vi "test-rotation3d.vi"(8 "error in (no error)":errorcluster) -> (0 "error out":errorcluster, 3 "ALL TESTS PASSED":bool)   [LabVIEW 2019]
uses:
  <vilib>/Rock Robotics/WPI/ThirdParty/JAS_Junk/TrajLib/TypeDef/ROTATION3D.ctl
  <vilib>/Rock Robotics/WPI/ThirdParty/JAS_Junk/TrajLib/TypeDef/QUATERNION.ctl
  <vilib>/Rock Robotics/WPI/ThirdParty/JAS_Junk/TrajLib/VI/Quaternion_New_Default.vi
  <vilib>/Rock Robotics/WPI/ThirdParty/JAS_Junk/TrajLib/MatBuilder_Create.vi
  <vilib>/Rock Robotics/WPI/ThirdParty/JAS_Junk/TrajLib/VI/Vector_Norm.vi
  <vilib>/Rock Robotics/WPI/ThirdParty/JAS_Junk/TrajLib/VI/Quaternion_New.vi
  <vilib>/Rock Robotics/WPI/ThirdParty/JAS_Junk/TrajLib/VecBuilder_ArrayBy1Fill.vi
  <vilib>/Rock Robotics/WPI/ThirdParty/JAS_Junk/TrajLib/VI/Quaternion_Equals.vi
  <vilib>/Rock Robotics/WPI/ThirdParty/JAS_Junk/TrajLib/VI/Vector_Dot.vi
  <vilib>/Rock Robotics/WPI/ThirdParty/JAS_Junk/TrajLib/VI/Rotation3d_Create_Quaternion.vi
  <vilib>/Analysis/7linalg.llb/QR Decomposition.vi
  <vilib>/Analysis/7linalg.llb/Real QR Decomposition.vi
  <vilib>/Rock Robotics/WPI/ThirdParty/JAS_Junk/TrajLib/Matrix_Transpose.vi
  <vilib>/Analysis/baseanly.llb/A x B.vi
  <vilib>/Analysis/baseanly.llb/Real A x B.vi
  <vilib>/Analysis/baseanly.llb/Determinant.vi
  <vilib>/Analysis/baseanly.llb/Real Determinant.vi
  <vilib>/Rock Robotics/WPI/ThirdParty/JAS_Junk/TrajLib/Matrix_NormF.vi
  <vilib>/Rock Robotics/WPI/ThirdParty/JAS_Junk/TrajLib/MatrixHelper_CoerceSize.vi
  <vilib>/Rock Robotics/WPI/ThirdParty/JAS_Junk/TrajLib/VI/Rotation3d_Times.vi
  <vilib>/Rock Robotics/WPI/ThirdParty/JAS_Junk/TrajLib/MathUtil_Clamp.vi
  <vilib>/Rock Robotics/WPI/ThirdParty/JAS_Junk/TrajLib/Util_CalcDist.vi
  <vilib>/Rock Robotics/WPI/ThirdParty/JAS_Junk/TrajLib/VI/Quaternion_Get_Vect.vi
  <vilib>/Rock Robotics/WPI/ThirdParty/JAS_Junk/TrajLib/VI/Quaternion_Get_W.vi
  <vilib>/Rock Robotics/WPI/ThirdParty/JAS_Junk/TrajLib/VI/Rotation3d_UnaryMinus.vi
  <vilib>/Rock Robotics/WPI/ThirdParty/JAS_Junk/TrajLib/VI/Quaternion_Times.vi
  <vilib>/Rock Robotics/WPI/ThirdParty/JAS_Junk/TrajLib/VI/Quaternion_Normalize.vi
  <vilib>/Analysis/_algsub.llb/Matrix Norm.vi
  <vilib>/Analysis/_algsub.llb/Real Matrix Norm.vi
  <vilib>/Rock Robotics/WPI/ThirdParty/JAS_Junk/TrajLib/VI/Quaternion_Inverse.vi
  <vilib>/Analysis/Matrix/Numeric/Conversions/Array To Matrix - RA.vi
  <vilib>/Analysis/7linalg.llb/Create Special Matrix.vi
  <vilib>/Analysis/7linalg.llb/Create Special Real Matrix.vi
  <vilib>/Analysis/Matrix/Numeric/Subtract/Subtract.vi
  <vilib>/Analysis/Matrix/Numeric/Subtract/Subtract - RM,RM.vi
  <vilib>/Analysis/Matrix/Numeric/Multiply/Multiply - RM,R.vi
  <vilib>/Rock Robotics/WPI/ThirdParty/JAS_Junk/TrajLib/Trajectory_Library.lvlib
  <vilib>/Analysis/Matrix/NI_Matrix.lvlib
panel:
  out "Axis Angle\nTest Passed":bool
  out "Two Vectors\nTest Passed":bool
  out "Rotation3d 2":T1={"Q_quaternion"={"R"=1.0, "V"=[0.0, 0.0, 0.0]}}
  out "Rotation3d":T1={"Q_quaternion"={"R"=1.0, "V"=[0.0, 0.0, 0.0]}}
  out "Rot Mat\nTest Passed":bool
  # "ROTATION3D TEST"
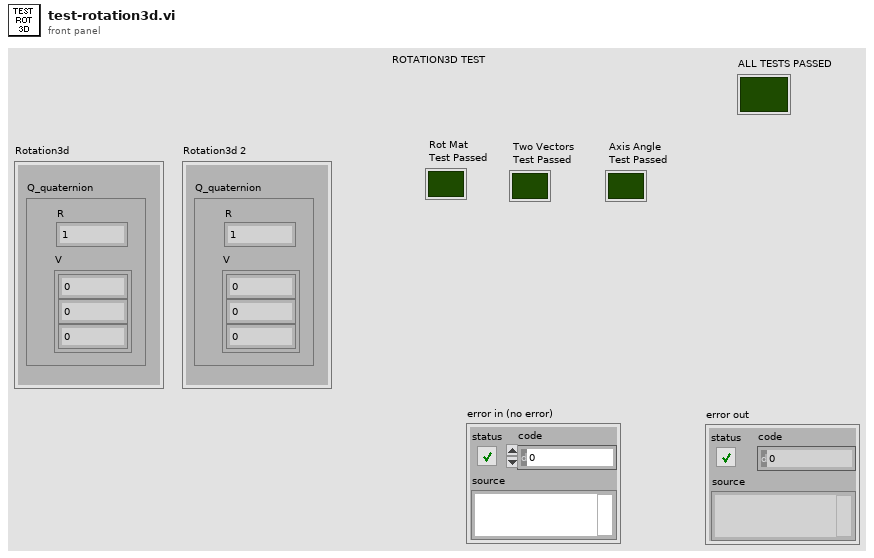
[diagram p1: front panel]
types:
  T1 = typedef "Trajectory_Library.lvlib/ROTATION3D.ctl" = cluster{"Q_quaternion":T2}
  T2 = typedef "Trajectory_Library.lvlib/QUATERNION.ctl" = cluster{"R":dbl, "V":dbl[]}
  T3 = typedef "NI_Matrix.lvlib/RealMatrix.ctl" = dbl[][]
  T4 = typedef "Trajectory_Library.lvlib/ROTATION2D.ctl" = cluster{"VALUE":dbl, "COS":dbl, "SIN":dbl}
diagram:
  w17 = 1.0  # R2
  w16 = 0.0  # R1
  w15 = 0.0  # R0
  w21 = 0.0  # R2
  w20 = 1.0  # R1
  w19 = 0.0  # R0
  w27 = 0.0  # R2
  w26 = 0.0  # R1
  w25 = 1.0  # R0
  w32 = 0.0  # Roll  Degrees
  w33 = 0.0  # Pitch  Degrees
  w34 = 60.0  # Yaw  Degrees
  w43 = 60.0  # Angle Degrees
  w41 = 1.0  # Z
  w39 = 0.0  # X
  w40 = 0.0  # Y
  w45 = 0.0  # Roll  Degrees
  w46 = 60.0  # Pitch  Degrees
  w47 = 0.0  # Yaw  Degrees
  w56 = 60.0  # Angle Degrees
  w54 = 0.0  # Z
  w52 = 0.0  # X
  w53 = 1.0  # Y
  w59 = 60.0  # Roll  Degrees
  w60 = 0.0  # Pitch  Degrees
  w61 = 0.0  # Yaw  Degrees
  w70 = 60.0  # Angle Degrees
  w68 = 0.0  # Z
  w66 = 1.0  # X
  w67 = 0.0  # Y
  w169 = 0.0  # z
  w168 = 1.0  # y
  w167 = 1.0  # x
  w181 = 1.0  # z
  w180 = 0.0  # y
  w179 = 0.0  # x
  w184 = 0.0  # z
  w183 = 1.0  # y
  w182 = 0.0  # x
  w187 = 0.0  # z
  w186 = 0.0  # y
  w185 = 1.0  # x
  w198 = 3  # Columns
  w197 = 3  # Rows
  w214 = 0.0  # Roll  Degrees
  w215 = 0.0  # Pitch  Degrees
  w216 = 90.0  # Yaw  Degrees
  w237 = 1.0  # R2
  w236 = 0.0  # R1
  w235 = 0.0  # R0
  w240 = 0.0  # R2
  w239 = 0.0  # R1
  w238 = -1.0  # R0
  w243 = 0.0  # R2
  w242 = 1.0  # R1
  w241 = 0.0  # R0
  # "final var rvec3 = new Rotation3d(zAxis.times(Math.PI / 3));\n    assertEquals(rot5, rvec3);"
  # "final var rvec2 = new Rotation3d(yAxis.times(Math.PI / 3));\n    assertEquals(rot3, rvec2);"
  # "final var rvec1 = new Rotation3d(xAxis.times(Math.PI / 3));\n    assertEquals(rot1, rvec1);"
  # "3d Rotation"
  # "3d Rotation"
  # "3d Rotation"
  # "3d Rotation"
  # "3d Rotation"
  # "3d Rotation"
  # "@Test\n  void testInitAxisAngleAndRollPitchYaw() {\n    final var xAxis = VecBuilder.fill(1.0, 0.0, 0.0);\n    final var rot1 = new Rotation3d(xAxis, Math.PI / 3);\n    final var rot2 = new Rotation3d(Math.PI / 3, 0.0, 0.0);\n    assertEquals(rot1, rot2);\n\n    final var yAxis = VecBuilder.fill(0.0, 1.0, 0.0);\n    final var rot3 = new Rotation3d(yAxis, Math.PI / 3);\n    final var rot4 = new Rotation3d(0.0, Math.PI / 3, 0.0);\n    assertEquals(rot3, rot4);\n\n    final var zAxis = VecBuilder.fill(0.0, 0.0, 1.0);\n    final var rot5 = new Rotation3d(zAxis, Math.PI / 3);\n    final var rot6 = new Rotation3d(0.0, 0.0, Math.PI / 3);\n    assertEquals(rot5, rot6);\n  }"
  # "180 degree rotation of z-axes"
  # "180 degree rotation of y-axes"
  # "180 degree rotation of x-axes"
  # "0 degree rotation of z-axes"
  # "0 degree rotation of y-axes"
  # "0 degree rotation of x-axes"
  # "45 degree CCW rotation around z-axis"
  # "90 degree CW rotation around y-axis"
  # "z"
  # "y"
  # "X"
  # "@Test\n  void testInitTwoVector() {\n    final var xAxis = VecBuilder.fill(1.0, 0.0, 0.0);\n    final var yAxis = VecBuilder.fill(0.0, 1.0, 0.0);\n    final var zAxis = VecBuilder.fill(0.0, 0.0, 1.0);\n\n    // 90 degree CW rotation around y-axis\n    final var rot1 = new Rotation3d(xAxis, zAxis);\n    final var expected1 = new Rotation3d(yAxis, -Math.PI / 2.0);\n    assertEquals(expected1, rot1);\n\n    // 45 degree CCW rotation around z-axis\n    final var rot2 = new Rotation3d(xAxis, VecBuilder.fill(1.0, 1.0, 0.0));\n    final var expected2 = new Rotation3d(zAxis, Math.PI / 4.0);\n    assertEquals(expected2, rot2);\n\n    // 0 degree rotation of x-axes\n    final var rot3 = new Rotation3d(xAxis, xAxis);\n    assertEquals(new Rotation3d(), rot3);\n\n    // 0 degree rotation of y-axes\n    final var rot4 = new Rotation3d(yAxis, yAxis);\n    assertEquals(new Rotation3d(), rot4);\n\n    // 0 degree rotation of z-axes\n    final var rot5 = new Rotation3d(zAxis, zAxis);\n    assertEquals(new Rotation3d(), rot5);\n\n    // 180 degree rotation tests. For 180 degree rotations, any quaternion with\n    // an orthogonal rotation axis is acceptable. The rotation axis and initial\n    // vector are orthogonal if their dot product is zero.\n\n    // 180 degree rotation of x-axes\n    final var rot6 = new Rotation3d(xAxis, xAxis.times(-1.0));\n    final var q6 = rot6.getQuaternion();\n    assertEquals(0.0, q6.getW());\n    assertEquals(\n        0.0,\n        q6.getX() * xAxis.get(0, 0) + q6.getY() * xAxis.get(1, 0) + q6.getZ() * xAxis.get(2, 0));\n\n    // 180 degree rotation of y-axes\n    final var rot7 = new Rotation3d(yAxis, yAxis.times(-1.0));\n    final var q7 = rot7.getQuaternion();\n    assertEquals(0.0, q7.getW());\n    assertEquals(\n        0.0,\n        q7.getX() * yAxis.get(0, 0) + q7.getY() * yAxis.get(1, 0) + q7.getZ() * yAxis.get(2, 0));\n\n    // 180 degree rotation of z-axes\n    final var rot8 = new Rotation3d(zAxis, zAxis.times(-1.0));\n    final var q8 = rot8.getQuaternion();\n    assertEquals(0.0, q8.getW());\n    assertEquals(\n        0.0,\n        q8.getX() * zAxis.get(0, 0) + q8.getY() * zAxis.get(1, 0) + q8.getZ() * zAxis.get(2, 0));\n  }"
  # "Matrix that's orthogonal but not special orthogonal"
  # "Matrix that isn't orthogonal"
  # "3d Rotation"
  # "90 degree CCW rotation around z-axis"
  # "@Test\n  void testInitRotationMatrix() {\n    // No rotation\n    final var R1 = Matrix.eye(Nat.N3());\n    final var rot1 = new Rotation3d(R1);\n    assertEquals(new Rotation3d(), rot1);\n\n    // 90 degree CCW rotation around z-axis\n    final var R2 = new Matrix<>(Nat.N3(), Nat.N3());\n    R2.assignBlock(0, 0, VecBuilder.fill(0.0, 1.0, 0.0));\n    R2.assignBlock(0, 1, VecBuilder.fill(-1.0, 0.0, 0.0));\n    R2.assignBlock(0, 2, VecBuilder.fill(0.0, 0.0, 1.0));\n    final var rot2 = new Rotation3d(R2);\n    final var expected2 = new Rotation3d(0.0, 0.0, Units.degreesToRadians(90.0));\n    assertEquals(expected2, rot2);\n\n    // Matrix that isn't orthogonal\n    final var R3 =\n        new MatBuilder<>(Nat.N3(), Nat.N3()).fill(1.0, 0.0, 0.0, 1.0, 0.0, 0.0, 1.0, 0.0, 0.0);\n    assertThrows(IllegalArgumentException.class, () -> new Rotation3d(R3));\n\n    // Matrix that's orthogonal but not special orthogonal\n    final var R4 = Matrix.eye(Nat.N3()).times(2.0);\n    assertThrows(IllegalArgumentException.class, () -> new Rotation3d(R4));\n  }"
  # "30 deg total\n7.5\n15\n22.5"
  # "// -160 minus half distance between 170 and -160 (15) = -175"
  # "// 50 + (70 - 50) * 0.5 = 60"
  # "30 deg total\n7.5\n15\n22.5"
  # "// -160 minus half distance between 170 and -160 (15) = -175"
  # "// 50 + (70 - 50) * 0.5 = 60"
  # "30 deg total\n7.5\n15\n22.5"
  # "// -160 minus half distance between 170 and -160 (15) = -175"
  # "// 50 + (70 - 50) * 0.5 = 60"
  # "// ===============================================================\n  @SuppressWarnings(\"LocalVariableName\")\n  @Test 16\n  void testInterpolate() {\n    final var xAxis = VecBuilder.fill(1.0, 0.0, 0.0);\n    final var yAxis = VecBuilder.fill(0.0, 1.0, 0.0);\n    final var zAxis = VecBuilder.fill(0.0, 0.0, 1.0);\n\n    // 50 + (70 - 50) * 0.5 = 60\n    var rot1 = new Rotation3d(xAxis, Units.degreesToRadians(50));\n    var rot2 = new Rotation3d(xAxis, Units.degreesToRadians(70));\n    var interpolated = rot1.interpolate(rot2, 0.5);\n    assertEquals(Units.degreesToRadians(60.0), interpolated.getX(), kEpsilon);\n    assertEquals(Units.degreesToRadians(0.0), interpolated.getY(), kEpsilon);\n    assertEquals(Units.degreesToRadians(0.0), interpolated.getZ(), kEpsilon);\n\n    // -160 minus half distance between 170 and -160 (15) = -175\n    rot1 = new Rotation3d(xAxis, Units.degreesToRadians(170));\n    rot2 = new Rotation3d(xAxis, Units.degreesToRadians(-160));\n    interpolated = rot1.interpolate(rot2, 0.5);\n    assertEquals(Units.degreesToRadians(-175.0), interpolated.getX());\n    assertEquals(Units.degreesToRadians(0.0), interpolated.getY(), kEpsilon);\n    assertEquals(Units.degreesToRadians(0.0), interpolated.getZ());\n\n    // 50 + (70 - 50) * 0.5 = 60\n    rot1 = new Rotation3d(yAxis, Units.degreesToRadians(50));\n    rot2 = new Rotation3d(yAxis, Units.degreesToRadians(70));\n    interpolated = rot1.interpolate(rot2, 0.5);\n    assertEquals(Units.degreesToRadians(0.0), interpolated.getX(), kEpsilon);\n    assertEquals(Units.degreesToRadians(60.0), interpolated.getY(), kEpsilon);\n    assertEquals(Units.degreesToRadians(0.0), interpolated.getZ(), kEpsilon);\n\n    // -160 minus half distance between 170 and -160 (165) = 5\n    rot1 = new Rotation3d(yAxis, Units.degreesToRadians(170));\n    rot2 = new Rotation3d(yAxis, Units.degreesToRadians(-160));\n    interpolated = rot1.interpolate(rot2, 0.5);\n    assertEquals(Units.degreesToRadians(180.0), interpolated.getX(), kEpsilon);\n    assertEquals(Units.degreesToRadians(-5.0), interpolated.getY(), kEpsilon);\n    assertEquals(Units.degreesToRadians(180.0), interpolated.getZ(), kEpsilon);\n\n    // 50 + (70 - 50) * 0.5 = 60\n    rot1 = new Rotation3d(zAxis, Units.degreesToRadians(50));\n    rot2 = new Rotation3d(zAxis, Units.degreesToRadians(70));\n    interpolated = rot1.interpolate(rot2, 0.5);\n    assertEquals(Units.degreesToRadians(0.0), interpolated.getX(), kEpsilon);\n    assertEquals(Units.degreesToRadians(0.0), interpolated.getY(), kEpsilon);\n    assertEquals(Units.degreesToRadians(60.0), interpolated.getZ(), kEpsilon);\n\n    // -160 minus half distance between 170 and -160 (15) = -175\n    rot1 = new Rotation3d(zAxis, Units.degreesToRadians(170));\n    rot2 = new Rotation3d(zAxis, Units.degreesToRadians(-160));\n    interpolated = rot1.interpolate(rot2, 0.5);\n    assertEquals(Units.degreesToRadians(0.0), interpolated.getX(), kEpsilon);\n    assertEquals(Units.degreesToRadians(0.0), interpolated.getY(), kEpsilon);\n    assertEquals(Units.degreesToRadians(-175.0), interpolated.getZ(), kEpsilon);\n  }"
  # "// ===============================================================\n  @Test 15\n  void testInequality() {\n    @SuppressWarnings(\"LocalVariableName\")\n    final var zAxis = VecBuilder.fill(0.0, 0.0, 1.0);\n\n    var rot1 = new Rotation3d(zAxis, Units.degreesToRadians(43.0));\n    var rot2 = new Rotation3d(zAxis, Units.degreesToRadians(43.5));\n    assertNotEquals(rot1, rot2);\n  }"
  # "// ===============================================================\n  @Test 14\n  void testToRotation2d() {\n    var rotation =\n        new Rotation3d(\n            Units.degreesToRadians(20.0),\n            Units.degreesToRadians(30.0),\n            Units.degreesToRadians(40.0));\n    var expected = new Rotation2d(Units.degreesToRadians(40.0));\n\n    assertEquals(expected, rotation.toRotation2d());\n  }"
  # "// ===============================================================\n  @SuppressWarnings(\"LocalVariableName\")\n  @Test 13\n  void testAxisAngle() {\n    final var xAxis = VecBuilder.fill(1.0, 0.0, 0.0);\n    final var yAxis = VecBuilder.fill(0.0, 1.0, 0.0);\n    final var zAxis = VecBuilder.fill(0.0, 0.0, 1.0);\n\n    var rot1 = new Rotation3d(xAxis, Units.degreesToRadians(90.0));\n    assertEquals(xAxis, rot1.getAxis());\n    assertEquals(Math.PI / 2.0, rot1.getAngle(), 1e-9);\n\n    var rot2 = new Rotation3d(yAxis, Units.degreesToRadians(45.0));\n    assertEquals(yAxis, rot2.getAxis());\n    assertEquals(Math.PI / 4.0, rot2.getAngle(), 1e-9);\n\n    var rot3 = new Rotation3d(zAxis, Units.degreesToRadians(60.0));\n    assertEquals(zAxis, rot3.getAxis());\n    assertEquals(Math.PI / 3.0, rot3.getAngle(), 1e-9);\n  }"
  # "// ===============================================================\n  @Test 12\n  void testEquality() {\n    @SuppressWarnings(\"LocalVariableName\")\n    final var zAxis = VecBuilder.fill(0.0, 0.0, 1.0);\n\n    var rot1 = new Rotation3d(zAxis, Units.degreesToRadians(43.0));\n    var rot2 = new Rotation3d(zAxis, Units.degreesToRadians(43.0));\n    assertEquals(rot1, rot2);\n\n    rot1 = new Rotation3d(zAxis, Units.degreesToRadians(-180.0));\n    rot2 = new Rotation3d(zAxis, Units.degreesToRadians(180.0));\n    assertEquals(rot1, rot2);\n  }"
  # "// ===============================================================\n  @Test 11\n  void testMinus() {\n    @SuppressWarnings(\"LocalVariableName\")\n    final var zAxis = VecBuilder.fill(0.0, 0.0, 1.0);\n\n    var rot1 = new Rotation3d(zAxis, Units.degreesToRadians(70.0));\n    var rot2 = new Rotation3d(zAxis, Units.degreesToRadians(30.0));\n\n    assertEquals(rot1.minus(rot2).getZ(), Units.degreesToRadians(40.0), kEpsilon);\n  }"
  # "// ===============================================================\n  @Test 10\n  void testRotateByNonZeroZ() {\n    @SuppressWarnings(\"LocalVariableName\")\n    final var zAxis = VecBuilder.fill(0.0, 0.0, 1.0);\n\n    var rot = new Rotation3d(zAxis, Units.degreesToRadians(90.0));\n    rot = rot.plus(new Rotation3d(zAxis, Units.degreesToRadians(30.0)));\n\n    var expected = new Rotation3d(zAxis, Units.degreesToRadians(120.0));\n    assertEquals(expected, rot);\n  }"
  # "// ===============================================================\n  @Test 9\n  void testRotateByNonZeroY() {\n    @SuppressWarnings(\"LocalVariableName\")\n    final var yAxis = VecBuilder.fill(0.0, 1.0, 0.0);\n\n    var rot = new Rotation3d(yAxis, Units.degreesToRadians(90.0));\n    rot = rot.plus(new Rotation3d(yAxis, Units.degreesToRadians(30.0)));\n\n    var expected = new Rotation3d(yAxis, Units.degreesToRadians(120.0));\n    assertEquals(expected, rot);\n  }"
  # "// ===============================================================\n  @Test 8\n  void testRotateByNonZeroX() {\n    @SuppressWarnings(\"LocalVariableName\")\n    final var xAxis = VecBuilder.fill(1.0, 0.0, 0.0);\n\n    var rot = new Rotation3d(xAxis, Units.degreesToRadians(90.0));\n    rot = rot.plus(new Rotation3d(xAxis, Units.degreesToRadians(30.0)));\n\n    var expected = new Rotation3d(xAxis, Units.degreesToRadians(120.0));\n    assertEquals(expected, rot);\n  }"
  # "// ===============================================================\n  @SuppressWarnings(\"LocalVariableName\")\n  @Test 7\n  void testRotateByFromZeroZ() {\n    final var zAxis = VecBuilder.fill(0.0, 0.0, 1.0);\n\n    final var zero = new Rotation3d();\n    var rotated = zero.rotateBy(new Rotation3d(zAxis, Units.degreesToRadians(90.0)));\n\n    var expected = new Rotation3d(zAxis, Units.degreesToRadians(90.0));\n    assertEquals(expected, rotated);\n  }"
  # "// ===============================================================\n  @SuppressWarnings(\"LocalVariableName\")\n  @Test 6\n  void testRotateByFromZeroY() {\n    final var yAxis = VecBuilder.fill(0.0, 1.0, 0.0);\n\n    final var zero = new Rotation3d();\n    var rotated = zero.rotateBy(new Rotation3d(yAxis, Units.degreesToRadians(90.0)));\n\n    var expected = new Rotation3d(yAxis, Units.degreesToRadians(90.0));\n    assertEquals(expected, rotated);\n  }"
  # "// ===============================================================\n  @SuppressWarnings(\"LocalVariableName\")\n  @Test 5\n  void testRotateByFromZeroX() {\n    final var xAxis = VecBuilder.fill(1.0, 0.0, 0.0);\n\n    final var zero = new Rotation3d();\n    var rotated = zero.rotateBy(new Rotation3d(xAxis, Units.degreesToRadians(90.0)));\n\n    var expected = new Rotation3d(xAxis, Units.degreesToRadians(90.0));\n    assertEquals(expected, rotated);\n  }"
  # "// ===============================================================\n  @SuppressWarnings(\"LocalVariableName\")\n  @Test 4\n  void testRotationLoop() {\n    var rot = new Rotation3d();\n\n    rot = rot.plus(new Rotation3d(Units.degreesToRadians(90.0), 0.0, 0.0));\n    var expected = new Rotation3d(Units.degreesToRadians(90.0), 0.0, 0.0);\n    assertEquals(expected, rot);\n\n    rot = rot.plus(new Rotation3d(0.0, Units.degreesToRadians(90.0), 0.0));\n    expected =\n        new Rotation3d(\n            VecBuilder.fill(1.0 / Math.sqrt(3), 1.0 / Math.sqrt(3), -1.0 / Math.sqrt(3)),\n            Units.degreesToRadians(120.0));\n    assertEquals(expected, rot);\n\n    rot = rot.plus(new Rotation3d(0.0, 0.0, Units.degreesToRadians(90.0)));\n    expected = new Rotation3d(0.0, Units.degreesToRadians(90.0), 0.0);\n    assertEquals(expected, rot);\n\n    rot = rot.plus(new Rotation3d(0.0, Units.degreesToRadians(-90.0), 0.0));\n    assertEquals(new Rotation3d(), rot);\n  }"
  # "// ===============================================================\n  @Test 3\n  void testRadiansAndDegrees() {\n    @SuppressWarnings(\"LocalVariableName\")\n    final var zAxis = VecBuilder.fill(0.0, 0.0, 1.0);\n\n    var rot1 = new Rotation3d(zAxis, Units.degreesToRadians(45.0));\n    assertAll(\n        () -> assertEquals(0.0, rot1.getX(), kEpsilon),\n        () -> assertEquals(0.0, rot1.getY(), kEpsilon),\n        () -> assertEquals(Math.PI / 4.0, rot1.getZ(), kEpsilon));\n\n    var rot2 = new Rotation3d(zAxis, Units.degreesToRadians(30.0));\n    assertAll(\n        () -> assertEquals(0.0, rot2.getX(), kEpsilon),\n        () -> assertEquals(0.0, rot2.getY(), kEpsilon),\n        () -> assertEquals(Math.PI / 6.0, rot2.getZ(), kEpsilon));\n  }"
  # "// ===============================================================\n  @Test 2\n  void testRadiansToDegrees() {\n    @SuppressWarnings(\"LocalVariableName\")\n    final var zAxis = VecBuilder.fill(0.0, 0.0, 1.0);\n\n    var rot1 = new Rotation3d(zAxis, Math.PI / 3);\n    assertAll(\n        () -> assertEquals(Units.degreesToRadians(0.0), rot1.getX(), kEpsilon),\n        () -> assertEquals(Units.degreesToRadians(0.0), rot1.getY(), kEpsilon),\n        () -> assertEquals(Units.degreesToRadians(60.0), rot1.getZ(), kEpsilon));\n\n    var rot2 = new Rotation3d(zAxis, Math.PI / 4);\n    assertAll(\n        () -> assertEquals(Units.degreesToRadians(0.0), rot2.getX(), kEpsilon),\n        () -> assertEquals(Units.degreesToRadians(0.0), rot2.getY(), kEpsilon),\n        () -> assertEquals(Units.degreesToRadians(45.0), rot2.getZ(), kEpsilon));\n  }"
  # "// ===============================================================\n  @Test 1\n  void testInit() {\n    @SuppressWarnings(\"LocalVariableName\")\n    var xAxis = VecBuilder.fill(1.0, 0.0, 0.0);\n    final var rot1 = new Rotation3d(xAxis, Math.PI / 3);\n    final var rot2 = new Rotation3d(Math.PI / 3, 0.0, 0.0);\n    assertEquals(rot1, rot2);\n\n    @SuppressWarnings(\"LocalVariableName\")\n    var yAxis = VecBuilder.fill(0.0, 1.0, 0.0);\n    final var rot3 = new Rotation3d(yAxis, Math.PI / 3);\n    final var rot4 = new Rotation3d(0.0, Math.PI / 3, 0.0);\n    assertEquals(rot3, rot4);\n\n    @SuppressWarnings(\"LocalVariableName\")\n    final var zAxis = VecBuilder.fill(0.0, 0.0, 1.0);\n    final var rot5 = new Rotation3d(zAxis, Math.PI / 3);\n    final var rot6 = new Rotation3d(0.0, 0.0, Math.PI / 3);\n    assertEquals(rot5, rot6);\n  }"
  n1 = Divide(x=3.141592653589793, y=3.0) -> (x/y=w13:dbl)
  n2 = call <vilib>:"VecBuilder_3x1Fill.vi"("R2"=w27, "R1"=w26, "R0"=w25) -> ("output matrix"=w24:T3)  [unwired: 8 in]
  n3 = call <vilib>:"VecBuilder_3x1Fill.vi"("R2"=w21, "R1"=w20, "R0"=w19) -> ("output matrix"=w18:T3)  [unwired: 8 in]
  n4 = call <vilib>:"VecBuilder_3x1Fill.vi"("R2"=w17, "R1"=w16, "R0"=w15) -> ("output matrix"=w14:T3)  [unwired: 8 in]
  n5 = call-poly <vilib>:"Multiply.vi"("Real Scalar c"=w13, "Real Matrix A"=w24) -> ("A * c"=w6:T3)
  n6 = call-poly <vilib>:"Multiply.vi"("Real Scalar c"=w13, "Real Matrix A"=w18) -> ("A * c"=w4:T3)
  n7 = call-poly <vilib>:"Multiply.vi"("Real Scalar c"=w13, "Real Matrix A"=w14) -> ("A * c"=w2:T3)
  n8 = call <vilib>:"Rotation3D_Create_RotVector.vi"("RotationVector"=w2) -> ("Rotation3d"=w1:T1)  [unwired: 9 in, 1 out]
  n9 = call <vilib>:"Rotation3D_Create_RotVector.vi"("RotationVector"=w4) -> ("Rotation3d"=w3:T1)  [unwired: 9 in, 1 out]
  n10 = call <vilib>:"Rotation3D_Create_RotVector.vi"("RotationVector"=w6) -> ("Rotation3d"=w5:T1)  [unwired: 9 in, 1 out]
  n11 = Square Root(x=3.0) -> (sqrt(x)=w705:dbl)
  n12 = call <vilib>:"VecBuilder_3x1Fill.vi"("R2"=w169, "R1"=w168, "R0"=w167) -> ("output matrix"=w166:T3)  [unwired: 8 in]
  n13 = Divide(x=1.0, y=w705) -> (x/y=w702:dbl)
  n14 = call <vilib>:"VecBuilder_3x1Fill.vi"("R2"=w187, "R1"=w186, "R0"=w185) -> ("output matrix"=w130:T3)  [unwired: 8 in]
  n15 = call <vilib>:"VecBuilder_3x1Fill.vi"("R2"=w184, "R1"=w183, "R0"=w182) -> ("output matrix"=w76:T3)  [unwired: 8 in]
  n16 = call <vilib>:"Conv_Deg_Radians.vi"("Degress"=90.0) -> ("Radians"=w712:dbl)  [unwired: 10 in]
  n17 = call <vilib>:"VecBuilder_3x1Fill.vi"("R2"=w181, "R1"=w180, "R0"=w179) -> ("output matrix"=w75:T3)  [unwired: 8 in]
  n18 = Divide(x=3.141592653589793, y=3.0) -> (x/y=w830:dbl)
  n19 = call <vilib>:"Conv_Deg_Radians.vi"("Degress"=90.0) -> ("Radians"=w722:dbl)  [unwired: 10 in]
  n20 = Divide(x=3.141592653589793, y=3.0) -> (x/y=w805:dbl)
  n21 = Build Array(1.0 ("element"), 0.0 ("element"), 0.0 ("element")) -> (w835:dbl[])
  n22 = call <vilib>:"Conv_Deg_Radians.vi"("Degress"=-90.0) -> ("Radians"=w683:dbl)  [unwired: 10 in]
  n23 = call <vilib>:"Conv_Deg_Radians.vi"("Degress"=90.0) -> ("Radians"=w695:dbl)  [unwired: 10 in]
  n24 = Divide(x=3.141592653589793, y=3.0) -> (x/y=w802:dbl)
  n25 = Negate(x=w702) -> (-x=w703:dbl)
  n26 = call <vilib>:"Conv_Deg_Radians.vi"("Degress"=90.0) -> ("Radians"=w691:dbl)  [unwired: 10 in]
  n27 = call <vilib>:"Matrix_Create.vi"("Columns"=3, "Rows"=3) -> ("output matrix"=w232:T3)  [unwired: 9 in]
  n28 = Build Array(0.0 ("element"), 1.0 ("element"), 0.0 ("element")) -> (w824:dbl[])
  n29 = Build Array(0.0 ("element"), 0.0 ("element"), 1.0 ("element")) -> (w658:dbl[])
  n30 = Build Array(0.0 ("element"), 1.0 ("element"), 0.0 ("element")) -> (w668:dbl[])
  n31 = Build Array(1.0 ("element"), 0.0 ("element"), 0.0 ("element")) -> (w383:dbl[])
  n32 = call <vilib>:"VecBuilder_3x1Fill.vi"("R2"=w243, "R1"=w242, "R0"=w241) -> ("output matrix"=w227:T3)  [unwired: 8 in]
  n33 = Build Array(0.0 ("element"), 1.0 ("element"), 0.0 ("element")) -> (w332:dbl[])
  n34 = Build Array(1.0 ("element"), 0.0 ("element"), 0.0 ("element")) -> (w678:dbl[])
  n35 = call <vilib>:"Conv_Deg_Radians.vi"("Degress"=90.0) -> ("Radians"=w656:dbl)  [unwired: 10 in]
  n36 = Build Array(1.0 ("element"), 0.0 ("element"), 0.0 ("element")) -> (w640:dbl[])
  n37 = call <vilib>:"Conv_Deg_Radians.vi"("Degress"=90.0) -> ("Radians"=w666:dbl)  [unwired: 10 in]
  n38 = Build Array(1.0 ("element"), 0.0 ("element"), 0.0 ("element")) -> (w648:dbl[])
  n39 = call <vilib>:"VecBuilder_3x1Fill.vi"("R2"=w237, "R1"=w236, "R0"=w235) -> ("output matrix"=w229:T3)  [unwired: 8 in]
  n40 = Build Array(0.0 ("element"), 1.0 ("element"), 0.0 ("element")) -> (w617:dbl[])
  n41 = Build Array(0.0 ("element"), 1.0 ("element"), 0.0 ("element")) -> (w625:dbl[])
  n42 = Build Array(1.0 ("element"), 0.0 ("element"), 0.0 ("element")) -> (w633:dbl[])
  n43 = Build Array(0.0 ("element"), 0.0 ("element"), 1.0 ("element")) -> (w255:dbl[])
  n44 = call <vilib>:"VecBuilder_3x1Fill.vi"("R2"=w240, "R1"=w239, "R0"=w238) -> ("output matrix"=w228:T3)  [unwired: 8 in]
  n45 = Build Array(0.0 ("element"), 1.0 ("element"), 0.0 ("element")) -> (w610:dbl[])
  n46 = Build Array(0.0 ("element"), 0.0 ("element"), 1.0 ("element")) -> (w815:dbl[])
  n47 = call <vilib>:"Conv_Deg_Radians.vi"("Degress"=90.0) -> ("Radians"=w676:dbl)  [unwired: 10 in]
  n48 = call <vilib>:"Conv_Deg_Radians.vi"("Degress"=90.0) -> ("Radians"=w638:dbl)  [unwired: 10 in]
  n49 = Divide(x=3.141592653589793, y=3.0) -> (x/y=w795:dbl)
  n50 = call <vilib>:"Conv_Deg_Radians.vi"("Degress"=30.0) -> ("Radians"=w646:dbl)  [unwired: 10 in]
  n51 = call <vilib>:"Conv_Deg_Radians.vi"("Degress"=90.0) -> ("Radians"=w615:dbl)  [unwired: 10 in]
  n52 = call <vilib>:"Matrix_Ident.vi"("Size"=3) -> ("output matrix"=w194:T3)  [unwired: 9 in, 1 out]
  n53 = call <vilib>:"Conv_Deg_Radians.vi"("Degress"=30.0) -> ("Radians"=w623:dbl)  [unwired: 10 in]
  n54 = Divide(x=3.141592653589793, y=4.0) -> (x/y=w776:dbl)
  n55 = call <vilib>:"Conv_Deg_Radians.vi"("Degress"=120.0) -> ("Radians"=w631:dbl)  [unwired: 10 in]
  n56 = call <vilib>:"Conv_Deg_Radians.vi"("Degress"=120.0) -> ("Radians"=w608:dbl)  [unwired: 10 in]
  n57 = Build Array(0.0 ("element"), 0.0 ("element"), 1.0 ("element")) -> (w594:dbl[])
  n58 = Build Array(0.0 ("element"), 0.0 ("element"), 1.0 ("element")) -> (w602:dbl[])
  n59 = Build Array(0.0 ("element"), 0.0 ("element"), 1.0 ("element")) -> (w587:dbl[])
  n60 = Build Array(0.0 ("element"), 0.0 ("element"), 1.0 ("element")) -> (w571:dbl[])
  n61 = Build Array(0.0 ("element"), 0.0 ("element"), 1.0 ("element")) -> (w550:dbl[])
  n62 = Build Array(0.0 ("element"), 0.0 ("element"), 1.0 ("element")) -> (w579:dbl[])
  n63 = Build Array(0.0 ("element"), 0.0 ("element"), 1.0 ("element")) -> (w556:dbl[])
  n64 = call <vilib>:"Conv_Deg_Radians.vi"("Degress"=90.0) -> ("Radians"=w592:dbl)  [unwired: 10 in]
  n65 = call <vilib>:"Conv_Deg_Radians.vi"("Degress"=30.0) -> ("Radians"=w600:dbl)  [unwired: 10 in]
  n66 = Build Array(0.0 ("element"), 0.0 ("element"), 1.0 ("element")) -> (w564:dbl[])
  n67 = Build Array(1.0 ("element"), 0.0 ("element"), 0.0 ("element")) -> (w512:dbl[])
  n68 = call <vilib>:"Conv_Deg_Radians.vi"("Degress"=120.0) -> ("Radians"=w585:dbl)  [unwired: 10 in]
  n69 = Build Array(0.0 ("element"), 0.0 ("element"), 1.0 ("element")) -> (w536:dbl[])
  n70 = Build Array(0.0 ("element"), 0.0 ("element"), 1.0 ("element")) -> (w542:dbl[])
  n71 = call <vilib>:"Conv_Deg_Radians.vi"("Degress"=70.0) -> ("Radians"=w569:dbl)  [unwired: 10 in]
  n72 = call <vilib>:"Conv_Deg_Radians.vi"("Degress"=43.0) -> ("Radians"=w548:dbl)  [unwired: 10 in]
  n73 = call <vilib>:"Conv_Deg_Radians.vi"("Degress"=30.0) -> ("Radians"=w577:dbl)  [unwired: 10 in]
  n74 = call <vilib>:"Conv_Deg_Radians.vi"("Degress"=43.0) -> ("Radians"=w554:dbl)  [unwired: 10 in]
  n75 = Build Array(0.0 ("element"), 1.0 ("element"), 0.0 ("element")) -> (w491:dbl[])
  n76 = call <vilib>:"Conv_Deg_Radians.vi"("Degress"=45.0) -> ("Radians"=w733:dbl)  [unwired: 10 in]
  n77 = Build Array(0.0 ("element"), 0.0 ("element"), 1.0 ("element")) -> (w798:dbl[])
  n78 = call <vilib>:"Conv_Deg_Radians.vi"("Degress"=40.0) -> ("Radians"=w562:dbl)  [unwired: 10 in]
  n79 = call <vilib>:"Conv_Deg_Radians.vi"("Degress"=-180.0) -> ("Radians"=w534:dbl)  [unwired: 10 in]
  n80 = Build Array(0.0 ("element"), 0.0 ("element"), 1.0 ("element")) -> (w779:dbl[])
  n81 = Build Array(0.0 ("element"), 0.0 ("element"), 1.0 ("element")) -> (w759:dbl[])
  n82 = call <vilib>:"Conv_Deg_Radians.vi"("Degress"=180.0) -> ("Radians"=w540:dbl)  [unwired: 10 in]
  n83 = Build Array(0.0 ("element"), 0.0 ("element"), 1.0 ("element")) -> (w490:dbl[])
  n84 = Build Array(0.0 ("element"), 0.0 ("element"), 1.0 ("element")) -> (w745:dbl[])
  n85 = Build Array(w702, w702, w703) -> (w710:dbl[])
  n86 = call <vilib>:"Rotation3d_Create_RollPitchYaw.vi"("Yaw"=0.0, "Pitch"=0.0, "Roll"=w722) -> ("Rotation3d"=w718:T1)  [unwired: 8 in]
  n87 = call <vilib>:"Conv_Deg_Radians.vi"("Degress"=30.0) -> ("Radians"=w728:dbl)  [unwired: 10 in]
  n88 = call <vilib>:"Rotation3d_Create_Default.vi"() -> ("ROTATION3D"=w719:T1)  [unwired: 11 in]
  n89 = call <vilib>:"Rotation3d_Create_RollPitchYaw.vi"("Yaw"=0.0, "Pitch"=w712, "Roll"=0.0 ("Pitch")) -> ("Rotation3d"=w714:T1)  [unwired: 8 in]
  n90 = call <vilib>:"Conv_Deg_Radians.vi"("Degress"=120.0) -> ("Radians"=w708:dbl)  [unwired: 10 in]
  n91 = call <vilib>:"Conv_Deg_Radians.vi"("Degress"=20.0) -> ("Radians"=w475:dbl)  [unwired: 10 in]
  n92 = Build Array(0.0 ("element"), 0.0 ("element"), 1.0 ("element")) -> (w466:dbl[])
  n93 = call <vilib>:"Conv_Deg_Radians.vi"("Degress"=30.0) -> ("Radians"=w474:dbl)  [unwired: 10 in]
  n94 = call <vilib>:"Conv_Deg_Radians.vi"("Degress"=40.0) -> ("Radians"=w473:dbl)  [unwired: 10 in]
  n95 = call <vilib>:"Conv_Deg_Radians.vi"("Degress"=40.0) -> ("Radians"=w471:dbl)  [unwired: 10 in]
  n96 = call <vilib>:"Conv_Deg_Radians.vi"("Degress"=43.0) -> ("Radians"=w464:dbl)  [unwired: 10 in]
  n97 = Build Array(0.0 ("element"), 0.0 ("element"), 1.0 ("element")) -> (w460:dbl[])
  n98 = call <vilib>:"Rotation3d_Create_RollPitchYaw.vi"("Yaw"=w695, "Pitch"=0.0 ("Yaw"), "Roll"=0.0 ("Pitch")) -> ("Rotation3d"=w699:T1)  [unwired: 8 in]
  n99 = call <vilib>:"Conv_Deg_Radians.vi"("Degress"=43.5) -> ("Radians"=w458:dbl)  [unwired: 10 in]
  n100 = Divide(x=3.141592653589793, y=4.0) -> (x/y=w730:dbl)
  n101 = call <vilib>:"Rotation3d_Create_AxisAngle.vi"("Angle"=w830, "Axis Vector"=w835) -> ("Rotation3d"=w829:T1)  [unwired: 9 in]
  n102 = call <vilib>:"Rotation3d_Create_RollPitchYaw.vi"("Yaw"=0.0, "Pitch"=w691, "Roll"=0.0 ("Pitch")) -> ("Rotation3d"=w690:T1)  [unwired: 8 in]
  n103 = call-poly <vilib>:"Multiply.vi"("Real Scalar c"=2.0, "Real Matrix A"=w194) -> ("A * c"=w192:T3)
  n104 = call <vilib>:"Rotation3d_Create_RollPitchYaw.vi"("Yaw"=0.0, "Pitch"=w683, "Roll"=0.0 ("Pitch")) -> ("Rotation3d"=w687:T1)  [unwired: 8 in]
  n105 = call <vilib>:"Rotation3d_Create_Default.vi"() -> ("ROTATION3D"=w651:T1)  [unwired: 11 in]
  n106 = call <vilib>:"Rotation3d_Create_RollPitchYaw.vi"("Yaw"=0.0, "Pitch"=0.0, "Roll"=w830) -> ("Rotation3d"=w828:T1)  [unwired: 8 in]
  n107 = call <vilib>:"Rotation3d_Create_Default.vi"() -> ("ROTATION3D"=w661:T1)  [unwired: 11 in]
  n108 = call <vilib>:"Rotation3d_Create_AxisAngle.vi"("Angle"=w805, "Axis Vector"=w824) -> ("Rotation3d"=w820:T1)  [unwired: 9 in]
  n109 = call <vilib>:"Rotation3d_Create_AxisAngle.vi"("Angle"=w656, "Axis Vector"=w658) -> ("Rotation3d"=w650:T1)  [unwired: 9 in]
  n110 = call <vilib>:"Rotation3d_Create_AxisAngle.vi"("Angle"=w666, "Axis Vector"=w668) -> ("Rotation3d"=w660:T1)  [unwired: 9 in]
  n111 = call <vilib>:"Rotation3d_Create_Default.vi"() -> ("ROTATION3D"=w672:T1)  [unwired: 11 in]
  n112 = call <vilib>:"Units_DegreesToRadians.vi"("Degrees"=w214) -> ("Radians"=w217:dbl)  [unwired: 10 in]
  n113 = call <vilib>:"Units_DegreesToRadians.vi"("Degrees"=w215) -> ("Radians"=w218:dbl)  [unwired: 10 in]
  n114 = call <vilib>:"Rotation3d_Create_AxisAngle.vi"("Angle"=w676, "Axis Vector"=w678) -> ("Rotation3d"=w670:T1)  [unwired: 9 in]
  n115 = call <vilib>:"Units_DegreesToRadians.vi"("Degrees"=w216) -> ("Radians"=w219:dbl)  [unwired: 10 in]
  n116 = Build Array(1.0 ("element"), 0.0 ("element"), 0.0 ("element"), 1.0 ("element"), 0.0 ("element"), 0.0 ("element"), 1.0 ("element"), 0.0 ("element"), 0.0 ("element")) -> (w208:dbl[])
  n117 = call <vilib>:"Rotation3d_Create_AxisAngle.vi"("Angle"=w638, "Axis Vector"=w640) -> ("Rotation3d"=w634:T1)  [unwired: 9 in]
  n118 = call <vilib>:"Rotation3d_Create_AxisAngle.vi"("Angle"=w646, "Axis Vector"=w648) -> ("Rotation3d"=w641:T1)  [unwired: 9 in]
  n119 = call <vilib>:"Rotation3d_Create_AxisAngle.vi"("Angle"=w615, "Axis Vector"=w617) -> ("Rotation3d"=w611:T1)  [unwired: 9 in]
  n120 = call <vilib>:"Rotation3d_Create_RollPitchYaw.vi"("Yaw"=0.0, "Pitch"=w805, "Roll"=0.0 ("Pitch")) -> ("Rotation3d"=w819:T1)  [unwired: 8 in]
  n121 = call <vilib>:"Rotation3d_Create_AxisAngle.vi"("Angle"=w623, "Axis Vector"=w625) -> ("Rotation3d"=w618:T1)  [unwired: 9 in]
  n122 = call <vilib>:"Rotation3d_Create_AxisAngle.vi"("Angle"=w631, "Axis Vector"=w633) -> ("Rotation3d"=w627:T1)  [unwired: 9 in]
  n123 = call <vilib>:"Rotation3d_Create_AxisAngle.vi"("Angle"=w608, "Axis Vector"=w610) -> ("Rotation3d"=w604:T1)  [unwired: 9 in]
  n124 = call <vilib>:"Rotation3d_Create_AxisAngle.vi"("Angle"=w802, "Axis Vector"=w815) -> ("Rotation3d"=w811:T1)  [unwired: 9 in]
  n125 = call <vilib>:"Rotation3d_Create_AxisAngle.vi"("Angle"=w592, "Axis Vector"=w594) -> ("Rotation3d"=w588:T1)  [unwired: 9 in]
  n126 = call <vilib>:"Rotation3d_Create_AxisAngle.vi"("Angle"=w600, "Axis Vector"=w602) -> ("Rotation3d"=w595:T1)  [unwired: 9 in]
  n127 = call <vilib>:"Rotation3d_Create_AxisAngle.vi"("Angle"=w585, "Axis Vector"=w587) -> ("Rotation3d"=w581:T1)  [unwired: 9 in]
  n128 = call <vilib>:"Rotation3d_Create_RollPitchYaw.vi"("Yaw"=w802, "Pitch"=0.0, "Roll"=0.0 ("Yaw")) -> ("Rotation3d"=w810:T1)  [unwired: 8 in]
  n129 = call <vilib>:"Rotation3d_Create_AxisAngle.vi"("Angle"=w569, "Axis Vector"=w571) -> ("Rotation3d"=w565:T1)  [unwired: 9 in]
  n130 = call <vilib>:"Rotation3d_Create_AxisAngle.vi"("Angle"=w548, "Axis Vector"=w550) -> ("Rotation3d"=w543:T1)  [unwired: 9 in]
  n131 = call <vilib>:"Rotation3d_Create_AxisAngle.vi"("Angle"=w577, "Axis Vector"=w579) -> ("Rotation3d"=w572:T1)  [unwired: 9 in]
  n132 = call <vilib>:"Rotation3d_Create_AxisAngle.vi"("Angle"=w554, "Axis Vector"=w556) -> ("Rotation3d"=w544:T1)  [unwired: 9 in]
  n133 = call <vilib>:"Rotation3d_Create_AxisAngle.vi"("Angle"=w562, "Axis Vector"=w564) -> ("Rotation3d"=w558:T1)  [unwired: 9 in]
  n134 = call <vilib>:"Rotation3d_Create_AxisAngle.vi"("Angle"=w534, "Axis Vector"=w536) -> ("Rotation3d"=w529:T1)  [unwired: 9 in]
  n135 = call <vilib>:"Rotation3d_Create_AxisAngle.vi"("Angle"=w540, "Axis Vector"=w542) -> ("Rotation3d"=w530:T1)  [unwired: 9 in]
  n136 = call <vilib>:"Rotation3d_Create_AxisAngle.vi"("Angle"=w795, "Axis Vector"=w798) -> ("Rotation3d"=w794:T1)  [unwired: 9 in]
  n137 = call "Matrix_ExtractCol_To_1D_Array.vi"("Input Matrix"=w76) -> ("Column Array"=w178:dbl[])  [unwired: 10 in]
  n138 = call <vilib>:"Rotation3d_Create_AxisAngle.vi"("Angle"=w776, "Axis Vector"=w779) -> ("Rotation3d"=w775:T1)  [unwired: 9 in]
  n139 = call <vilib>:"Rotation3d_Create_AxisAngle.vi"("Angle"=w733, "Axis Vector"=w759) -> ("Rotation3d"=w758:T1)  [unwired: 9 in]
  n140 = call <vilib>:"Rotation3d_Plus.vi"("other Rotation3d"=w718, "in Rotation3d"=w719) -> ("out Rotation3d"=w711:T1)  [unwired: 9 in]
  n141 = call <vilib>:"Rotation3d_Create_AxisAngle.vi"("Angle"=w728, "Axis Vector"=w745) -> ("Rotation3d"=w744:T1)  [unwired: 9 in]
  n142 = call <vilib>:"Rotation3d_Plus.vi"("other Rotation3d"=w714, "in Rotation3d"=w711) -> ("out Rotation3d"=w697:T1)  [unwired: 9 in]
  n143 = call "Matrix_ExtractCol_To_1D_Array.vi"("Input Matrix"=w75) -> ("Column Array"=w172:dbl[])  [unwired: 10 in]
  n144 = call <vilib>:"Rotation3d_Create_AxisAngle.vi"("Angle"=w708, "Axis Vector"=w710) -> ("Rotation3d"=w707:T1)  [unwired: 9 in]
  n145 = call <vilib>:"Matrix_AssignBlock.vi"("StartColumn"=0, "StartRow"=0, "Other Matrix"=w227, "input matrix"=w232) -> ("output matrix"=w231:T3)  [unwired: 7 in]
  n146 = call <vilib>:"Matrix_AssignBlock.vi"("StartColumn"=1, "StartRow"=0, "Other Matrix"=w228, "input matrix"=w231) -> ("output matrix"=w230:T3)  [unwired: 7 in]
  n147 = call <vilib>:"Matrix_AssignBlock.vi"("StartColumn"=2, "StartRow"=0, "Other Matrix"=w229, "input matrix"=w230) -> ("output matrix"=w220:T3)  [unwired: 7 in]
  n148 = call <vilib>:"Rotation3d_Create_AxisAngle.vi"("Angle"=w464, "Axis Vector"=w466) -> ("Rotation3d"=w454:T1)  [unwired: 9 in]
  n149 = call <vilib>:"Rotation3d_Plus.vi"("other Rotation3d"=w699, "in Rotation3d"=w697) -> ("out Rotation3d"=w685:T1)  [unwired: 9 in]
  n150 = call-poly <vilib>:"Multiply.vi"("Real Scalar c"=-1.0 ("y"), "Real Matrix A"=w76) -> ("A * c"=w125:T3)
  n151 = call <vilib>:"Rotation3d_Create_AxisAngle.vi"("Angle"=w458, "Axis Vector"=w460) -> ("Rotation3d"=w453:T1)  [unwired: 9 in]
  n152 = call-poly <vilib>:"Multiply.vi"("Real Scalar c"=-1.0 ("y"), "Real Matrix A"=w130) -> ("A * c"=w151:T3)
  n153 = call-poly <vilib>:"Multiply.vi"("Real Scalar c"=-1.0 ("y"), "Real Matrix A"=w75) -> ("A * c"=w100:T3)
  n154 = call <vilib>:"Rotation3d_Create_Default.vi"() -> ("ROTATION3D"=w681:T1)  [unwired: 11 in]
  n155 = call <vilib>:"Rotation3d_RotateBy.vi"("other Rotation3d"=w650, "in Rotation3d"=w651) -> ("out Rotation3d"=w652:T1)  [unwired: 9 in]
  n156 = call <vilib>:"Rotation3d_Plus.vi"("other Rotation3d"=w687, "in Rotation3d"=w685) -> ("out Rotation3d"=w682:T1)  [unwired: 9 in]
  n157 = call <vilib>:"Rotation3d_RotateBy.vi"("other Rotation3d"=w660, "in Rotation3d"=w661) -> ("out Rotation3d"=w662:T1)  [unwired: 9 in]
  n158 = call <vilib>:"Rotation3d_Create_RollPitchYaw.vi"("Yaw"=w219, "Pitch"=w218, "Roll"=w217) -> ("Rotation3d"=w212:T1)  [unwired: 8 in]
  "Rotation3d 2" <- w212
  n159 = call <vilib>:"Rotation3d_RotateBy.vi"("other Rotation3d"=w670, "in Rotation3d"=w672) -> ("out Rotation3d"=w671:T1)  [unwired: 9 in]
  n160 = call <vilib>:"Rotation3d_Create_RollPitchYaw.vi"("Yaw"=w473, "Pitch"=w474, "Roll"=w475) -> ("Rotation3d"=w470:T1)  [unwired: 8 in]
  n161 = call <vilib>:"Rotation3d_Plus.vi"("other Rotation3d"=w641, "in Rotation3d"=w634) -> ("out Rotation3d"=w642:T1)  [unwired: 9 in]
  n162 = call <vilib>:"Rotation3d_Plus.vi"("other Rotation3d"=w618, "in Rotation3d"=w611) -> ("out Rotation3d"=w619:T1)  [unwired: 9 in]
  n163 = call <vilib>:"Rotation2d_CreateAngle.vi"("Angle"=w471) -> ("ROTATION"=w468:T4)  [unwired: 10 in]
  n164 = call <vilib>:"Rotation3d_Equals.vi"("other Rotation3d"=w828, "in Rotation3d"=w829) -> ("Equals"=w809:bool)  [unwired: 9 in]
  n165 = call <vilib>:"Rotation3d_GetXYZ.vi"("in Rotation3d"=w794) -> ("Z"=w786:dbl, "Y"=w787:dbl, "X"=w788:dbl)  [unwired: 8 in]
  n166 = call <vilib>:"Conv_Deg_Radians.vi"("Degress"=60.0) -> ("Radians"=w784:dbl)  [unwired: 10 in]
  n167 = Divide(x=3.141592653589793, y=4.0) -> (x/y=w163:dbl)
  n168 = call <vilib>:"Rotation3d_GetXYZ.vi"("in Rotation3d"=w775) -> ("Z"=w767:dbl, "Y"=w768:dbl, "X"=w769:dbl)  [unwired: 8 in]
  n169 = call <vilib>:"Rotation3d_GetXYZ.vi"("in Rotation3d"=w758) -> ("Z"=w750:dbl, "Y"=w751:dbl, "X"=w752:dbl)  [unwired: 8 in]
  n170 = Negate(x=1.5707963267948966) -> (-x=w176:dbl)
  n171 = call <vilib>:"Conv_Deg_Radians.vi"("Degress"=45.0) -> ("Radians"=w765:dbl)  [unwired: 10 in]
  n172 = Divide(x=3.141592653589793, y=6.0) -> (x/y=w725:dbl)
  n173 = call <vilib>:"Rotation3d_Plus.vi"("other Rotation3d"=w595, "in Rotation3d"=w588) -> ("out Rotation3d"=w596:T1)  [unwired: 9 in]
  n174 = call <vilib>:"Rotation3d_GetXYZ.vi"("in Rotation3d"=w744) -> ("Z"=w736:dbl, "Y"=w737:dbl, "X"=w738:dbl)  [unwired: 8 in]
  n175 = call <vilib>:"Rotation3d_Equals.vi"("other Rotation3d"=w819, "in Rotation3d"=w820) -> ("Equals"=w808:bool)  [unwired: 9 in]
  n176 = call <vilib>:"Rotation3d_Minus.vi"("other Rotation3d"=w572, "in Rotation3d"=w565) -> ("out Rotation3d"=w573:T1)  [unwired: 9 in]
  n177 = call <vilib>:"Conv_Deg_Radians.vi"("Degress"=90.0) -> ("Radians"=w515:dbl)  [unwired: 10 in]
  n178 = call <vilib>:"Conv_Deg_Radians.vi"("Degress"=45.0) -> ("Radians"=w504:dbl)  [unwired: 10 in]
  n179 = call <vilib>:"Conv_Deg_Radians.vi"("Degress"=60.0) -> ("Radians"=w497:dbl)  [unwired: 10 in]
  n180 = call <vilib>:"Rotation3d_Equals.vi"("other Rotation3d"=w810, "in Rotation3d"=w811) -> ("Equals"=w807:bool)  [unwired: 9 in]
  n181 = call <vilib>:"Rotation3D_Create_RotMatrix.vi"("RotationMatrix"=w220) -> ("Error"=w209:bool, "Rotation3d"=w213:T1)  [unwired: 9 in]
  "Rotation3d" <- w213
  n182 = call <vilib>:"MatBuilder_Fill.vi"("Columns"=w198, "Rows"=w197, "Value List"=w208) -> ("output matrix"=w196:T3)  [unwired: 8 in]
  n183 = call <vilib>:"Rotation3d_Create_InitialFinalVector.vi"("Final Vector"=w75, "Initial Vector"=w130) -> ("ROTATION3D"=w175:T1)  [unwired: 9 in]
  n184 = call <vilib>:"Rotation3d_Create_AxisAngle.vi"("Angle"=w176, "Axis Vector"=w178) -> ("Rotation3d"=w174:T1)  [unwired: 9 in]
  n185 = Build Array(w52, w53, w54) -> (w51:dbl[])
  n186 = call <vilib>:"Rotation3d_Create_InitialFinalVector.vi"("Final Vector"=w125, "Initial Vector"=w76) -> ("ROTATION3D"=w124:T1)  [unwired: 9 in]
  n187 = Index Array(array=w76, index (row)=0, index (col)=0) -> (element=w104:dbl)
  n188 = Index Array(array=w76, index (row)=1, index (col)=0) -> (element=w103:dbl)
  n189 = call <vilib>:"Rotation3d_Equals.vi"("other Rotation3d"=w718, "in Rotation3d"=w711) -> ("Equals"=w717:bool)  [unwired: 9 in]
  n190 = call <vilib>:"Rotation3d_Create_InitialFinalVector.vi"("Final Vector"=w166, "Initial Vector"=w130) -> ("ROTATION3D"=w171:T1)  [unwired: 9 in]
  n191 = call <vilib>:"Rotation3d_Create_AxisAngle.vi"("Angle"=w163, "Axis Vector"=w172) -> ("Rotation3d"=w170:T1)  [unwired: 9 in]
  n192 = call <vilib>:"Rotation3d_Create_InitialFinalVector.vi"("Final Vector"=w151, "Initial Vector"=w130) -> ("ROTATION3D"=w150:T1)  [unwired: 9 in]
  n193 = Index Array(array=w130, index (row)=0, index (col)=0) -> (element=w129:dbl)
  n194 = call <vilib>:"Rotation3d_Equals.vi"("other Rotation3d"=w707, "in Rotation3d"=w697) -> ("Equals"=w701:bool)  [unwired: 9 in]
  n195 = call <vilib>:"Rotation3d_Equals.vi"("other Rotation3d"=w650, "in Rotation3d"=w652) -> ("Equals"=w649:bool)  [unwired: 9 in]
  n196 = Index Array(array=w130, index (row)=1, index (col)=0) -> (element=w128:dbl)
  n197 = call <vilib>:"Rotation3d_Equals.vi"("other Rotation3d"=w660, "in Rotation3d"=w662) -> ("Equals"=w659:bool)  [unwired: 9 in]
  n198 = Build Array(w39, w40, w41) -> (w38:dbl[])
  n199 = call <vilib>:"Rotation3d_Create_Default.vi"() -> ("ROTATION3D"=w157:T1)  [unwired: 11 in]
  n200 = Index Array(array=w76, index (row)=2, index (col)=0) -> (element=w102:dbl)
  n201 = call <vilib>:"Rotation3d_Create_InitialFinalVector.vi"("Final Vector"=w100, "Initial Vector"=w75) -> ("ROTATION3D"=w99:T1)  [unwired: 9 in]
  n202 = Index Array(array=w75, index (row)=0, index (col)=0) -> (element=w79:dbl)
  n203 = call <vilib>:"Rotation3d_Create_Default.vi"() -> ("ROTATION3D"=w160:T1)  [unwired: 11 in]
  n204 = call <vilib>:"Rotation3d_Create_InitialFinalVector.vi"("Final Vector"=w76, "Initial Vector"=w76) -> ("ROTATION3D"=w158:T1)  [unwired: 9 in]
  n205 = call <vilib>:"Rotation3d_Create_InitialFinalVector.vi"("Final Vector"=w130, "Initial Vector"=w130) -> ("ROTATION3D"=w161:T1)  [unwired: 9 in]
  n206 = Index Array(array=w75, index (row)=1, index (col)=0) -> (element=w78:dbl)
  n207 = call <vilib>:"Conv_Deg_Radians.vi"("Degress"=w56) -> ("Radians"=w55:dbl)  [unwired: 10 in]
  n208 = call <vilib>:"Rotation3d_Create_Default.vi"() -> ("ROTATION3D"=w155:T1)  [unwired: 11 in]
  n209 = Index Array(array=w130, index (row)=2, index (col)=0) -> (element=w127:dbl)
  n210 = call <vilib>:"Units_DegreesToRadians.vi"("Degrees"=w45) -> ("Radians"=w48:dbl)  [unwired: 10 in]
  n211 = call <vilib>:"Units_DegreesToRadians.vi"("Degrees"=w46) -> ("Radians"=w49:dbl)  [unwired: 10 in]
  n212 = call <vilib>:"Rotation3d_Equals.vi"("other Rotation3d"=w670, "in Rotation3d"=w671) -> ("Equals"=w669:bool)  [unwired: 9 in]
  n213 = call <vilib>:"Rotation3d_Create_InitialFinalVector.vi"("Final Vector"=w75, "Initial Vector"=w75) -> ("ROTATION3D"=w156:T1)  [unwired: 9 in]
  n214 = call <vilib>:"Units_DegreesToRadians.vi"("Degrees"=w47) -> ("Radians"=w50:dbl)  [unwired: 10 in]
  n215 = call <vilib>:"Rotation3d_Equals.vi"("other Rotation3d"=w627, "in Rotation3d"=w642) -> ("Equals"=w626:bool)  [unwired: 9 in]
  n216 = call <vilib>:"Rotation3d_Equals.vi"("other Rotation3d"=w604, "in Rotation3d"=w619) -> ("Equals"=w603:bool)  [unwired: 9 in]
  n217 = Index Array(array=w75, index (row)=2, index (col)=0) -> (element=w77:dbl)
  n218 = call <vilib>:"Conv_Deg_Radians.vi"("Degress"=w43) -> ("Radians"=w42:dbl)  [unwired: 10 in]
  n219 = call <vilib>:"Units_DegreesToRadians.vi"("Degrees"=w32) -> ("Radians"=w35:dbl)  [unwired: 10 in]
  n220 = call <vilib>:"Units_DegreesToRadians.vi"("Degrees"=w33) -> ("Radians"=w36:dbl)  [unwired: 10 in]
  n221 = call <vilib>:"Rotation3d_ToRotation2d.vi"("in Rotation3d"=w470) -> ("out Rotation2d"=w469:T4)  [unwired: 10 in]
  n222 = call <vilib>:"Units_DegreesToRadians.vi"("Degrees"=w34) -> ("Radians"=w37:dbl)  [unwired: 10 in]
  n223 = call <vilib>:"Rotation3d_Equals.vi"("other Rotation3d"=w681, "in Rotation3d"=w682) -> ("Equals"=w680:bool)  [unwired: 9 in]
  n224 = call <vilib>:"Rotation3d_Equals.vi"("other Rotation3d"=w690, "in Rotation3d"=w685) -> ("Equals"=w689:bool)  [unwired: 9 in]
  n225 = call <vilib>:"Rotation3d_Equals.vi"("other Rotation3d"=w581, "in Rotation3d"=w596) -> ("Equals"=w580:bool)  [unwired: 9 in]
  n226 = call <vilib>:"Rotation3d_Equals.vi"("other Rotation3d"=w453, "in Rotation3d"=w454) -> ("Equals"=w452:bool)  [unwired: 9 in]
  n227 = call <vilib>:"Rotation3d_Equals.vi"("other Rotation3d"=w558, "in Rotation3d"=w573) -> ("Equals"=w557:bool)  [unwired: 9 in]
  n228 = call <vilib>:"Rotation3d_Equals.vi"("other Rotation3d"=w544, "in Rotation3d"=w543) -> ("Equals"=w528:bool)  [unwired: 9 in]
  n229 = call <vilib>:"Conv_Deg_Radians.vi"("Degress"=50.0) -> ("Radians"=w440:dbl)  [unwired: 10 in]
  n230 = call <vilib>:"Conv_Deg_Radians.vi"("Degress"=70.0) -> ("Radians"=w438:dbl)  [unwired: 10 in]
  n231 = call <vilib>:"Rotation3d_Equals.vi"("other Rotation3d"=w530, "in Rotation3d"=w529) -> ("Equals"=w527:bool)  [unwired: 9 in]
  n232 = Build Array(w66, w67, w68) -> (w65:dbl[])
  n233 = call <vilib>:"Conv_Deg_Radians.vi"("Degress"=170.0) -> ("Radians"=w410:dbl)  [unwired: 10 in]
  n234 = call <vilib>:"Conv_Deg_Radians.vi"("Degress"=-160.0) -> ("Radians"=w408:dbl)  [unwired: 10 in]
  n235 = call <vilib>:"Conv_Deg_Radians.vi"("Degress"=50.0) -> ("Radians"=w379:dbl)  [unwired: 10 in]
  n236 = call <vilib>:"Conv_Deg_Radians.vi"("Degress"=70.0) -> ("Radians"=w377:dbl)  [unwired: 10 in]
  n237 = call <vilib>:"Conv_Deg_Radians.vi"("Degress"=w70) -> ("Radians"=w69:dbl)  [unwired: 10 in]
  n238 = call <vilib>:"Units_DegreesToRadians.vi"("Degrees"=w59) -> ("Radians"=w62:dbl)  [unwired: 10 in]
  n239 = call <vilib>:"Units_DegreesToRadians.vi"("Degrees"=w60) -> ("Radians"=w63:dbl)  [unwired: 10 in]
  n240 = call <vilib>:"Units_DegreesToRadians.vi"("Degrees"=w61) -> ("Radians"=w64:dbl)  [unwired: 10 in]
  n241 = call <vilib>:"Rotation3d_GetQuaterion.vi"("in Rotation3d"=w124) -> ("out Quaterion"=w122:T2)  [unwired: 10 in]
  n242 = call <vilib>:"Rotation3d_GetQuaterion.vi"("in Rotation3d"=w150) -> ("out Quaterion"=w148:T2)  [unwired: 10 in]
  n243 = call <vilib>:"Rotation3d_Create_AxisAngle.vi"("Angle"=w515, "Axis Vector"=w512) -> ("Rotation3d"=w514:T1)  [unwired: 9 in]
  n244 = call <vilib>:"Conv_Deg_Radians.vi"("Degress"=170.0) -> ("Radians"=w354:dbl)  [unwired: 10 in]
  n245 = call <vilib>:"Conv_Deg_Radians.vi"("Degress"=-160.0) -> ("Radians"=w352:dbl)  [unwired: 10 in]
  n246 = call <vilib>:"Rotation3d_Create_AxisAngle.vi"("Angle"=w504, "Axis Vector"=w491) -> ("Rotation3d"=w503:T1)  [unwired: 9 in]
  n247 = call <vilib>:"Rotation3d_GetQuaterion.vi"("in Rotation3d"=w99) -> ("out Quaterion"=w97:T2)  [unwired: 10 in]
  n248 = call <vilib>:"Rotation3D_Create_RotMatrix.vi"("RotationMatrix"=w196) -> ("Error"=w189:bool)  [unwired: 9 in, 1 out]
  n249 = call <vilib>:"Rotation3D_Create_RotMatrix.vi"("RotationMatrix"=w192) -> ("Error"=w188:bool)  [unwired: 9 in, 1 out]
  n250 = call <vilib>:"Rotation3d_Create_AxisAngle.vi"("Angle"=w497, "Axis Vector"=w490) -> ("Rotation3d"=w496:T1)  [unwired: 9 in]
  n251 = call <vilib>:"Conv_Deg_Radians.vi"("Degress"=50.0) -> ("Radians"=w314:dbl)  [unwired: 10 in]
  n252 = call <vilib>:"Conv_Deg_Radians.vi"("Degress"=70.0) -> ("Radians"=w312:dbl)  [unwired: 10 in]
  n253 = call <vilib>:"Rotation3d_Create_AxisAngle.vi"("Angle"=w55, "Axis Vector"=w51) -> ("Rotation3d"=w11:T1)  [unwired: 9 in]
  n254 = call <vilib>:"Conv_Deg_Radians.vi"("Degress"=170.0) -> ("Radians"=w289:dbl)  [unwired: 10 in]
  n255 = call <vilib>:"Conv_Deg_Radians.vi"("Degress"=-160.0) -> ("Radians"=w287:dbl)  [unwired: 10 in]
  n256 = call <vilib>:"Rotation3d_Create_AxisAngle.vi"("Angle"=w42, "Axis Vector"=w38) -> ("Rotation3d"=w10:T1)  [unwired: 9 in]
  n257 = call <vilib>:"Rotation3d_Equals.vi"("other Rotation3d"=w212, "in Rotation3d"=w213) -> ("Equals"=w211:bool)  [unwired: 9 in]
  n258 = Not(x=w209) -> (.not. x?=w210:bool)
  n259 = call <vilib>:"Rotation3d_Equals.vi"("other Rotation3d"=w174, "in Rotation3d"=w175) -> ("Equals"=w173:bool)  [unwired: 9 in]
  n260 = call <vilib>:"Util_ApproxEquals.vi"("Value 2"=0.0, "Value 1"=w787) -> ("ApproxEquals"=w790:bool)  [unwired: 9 in]
  n261 = call <vilib>:"Util_ApproxEquals.vi"("Value 2"=w784, "Value 1"=w786) -> ("ApproxEquals"=w789:bool)  [unwired: 9 in]
  n262 = call <vilib>:"Util_ApproxEquals.vi"("Value 2"=0.0, "Value 1"=w788) -> ("ApproxEquals"=w791:bool)  [unwired: 9 in]
  n263 = Compound Arithmetic op=AND(w809, w808, w807) -> (w806:bool)
  n264 = call <vilib>:"Rotation3d_Equals.vi"("other Rotation3d"=w170, "in Rotation3d"=w171) -> ("Equals"=w162:bool)  [unwired: 9 in]
  n265 = call <vilib>:"Util_ApproxEquals.vi"("Value 2"=0.0, "Value 1"=w768) -> ("ApproxEquals"=w771:bool)  [unwired: 9 in]
  n266 = call <vilib>:"Util_ApproxEquals.vi"("Value 2"=w765, "Value 1"=w767) -> ("ApproxEquals"=w770:bool)  [unwired: 9 in]
  n267 = call <vilib>:"Util_ApproxEquals.vi"("Value 2"=0.0, "Value 1"=w751) -> ("ApproxEquals"=w754:bool)  [unwired: 9 in]
  n268 = call <vilib>:"Util_ApproxEquals.vi"("Value 2"=w730, "Value 1"=w750) -> ("ApproxEquals"=w753:bool)  [unwired: 9 in]
  n269 = call <vilib>:"Util_ApproxEquals.vi"("Value 2"=0.0, "Value 1"=w769) -> ("ApproxEquals"=w772:bool)  [unwired: 9 in]
  n270 = call <vilib>:"Util_ApproxEquals.vi"("Value 2"=0.0, "Value 1"=w752) -> ("ApproxEquals"=w755:bool)  [unwired: 9 in]
  n271 = call <vilib>:"Util_ApproxEquals.vi"("Value 2"=0.0, "Value 1"=w737) -> ("ApproxEquals"=w740:bool)  [unwired: 9 in]
  n272 = call <vilib>:"Util_ApproxEquals.vi"("Value 2"=w725, "Value 1"=w736) -> ("ApproxEquals"=w739:bool)  [unwired: 9 in]
  n273 = call <vilib>:"Util_ApproxEquals.vi"("Value 2"=0.0, "Value 1"=w738) -> ("ApproxEquals"=w741:bool)  [unwired: 9 in]
  n274 = call <vilib>:"Rotation3d_Equals.vi"("other Rotation3d"=w157, "in Rotation3d"=w158) -> ("Equals"=w154:bool)  [unwired: 9 in]
  n275 = call <vilib>:"Rotation3d_Equals.vi"("other Rotation3d"=w160, "in Rotation3d"=w161) -> ("Equals"=w159:bool)  [unwired: 9 in]
  n276 = call <vilib>:"Rotation3d_Create_AxisAngle.vi"("Angle"=w440, "Axis Vector"=w383) -> ("Rotation3d"=w434:T1)  [unwired: 9 in]
  n277 = call <vilib>:"Rotation3d_Create_AxisAngle.vi"("Angle"=w438, "Axis Vector"=w383) -> ("Rotation3d"=w433:T1)  [unwired: 9 in]
  n278 = call <vilib>:"Rotation3d_Create_RollPitchYaw.vi"("Yaw"=w50, "Pitch"=w49, "Roll"=w48) -> ("Rotation3d"=w44:T1)  [unwired: 8 in]
  n279 = call <vilib>:"Rotation3d_Equals.vi"("other Rotation3d"=w155, "in Rotation3d"=w156) -> ("Equals"=w153:bool)  [unwired: 9 in]
  n280 = call <vilib>:"Rotation3d_Create_RollPitchYaw.vi"("Yaw"=w37, "Pitch"=w36, "Roll"=w35) -> ("Rotation3d"=w31:T1)  [unwired: 8 in]
  n281 = call <vilib>:"Rotation3d_Create_AxisAngle.vi"("Angle"=w410, "Axis Vector"=w383) -> ("Rotation3d"=w404:T1)  [unwired: 9 in]
  n282 = call <vilib>:"Rotation3d_Create_AxisAngle.vi"("Angle"=w408, "Axis Vector"=w383) -> ("Rotation3d"=w403:T1)  [unwired: 9 in]
  n283 = call <vilib>:"Rotation2d_Equals.vi"("other ROTATION"=w468, "in ROTATION"=w469) -> ("Equals"=w467:bool)  [unwired: 9 in]
  n284 = call <vilib>:"Rotation3d_Create_AxisAngle.vi"("Angle"=w69, "Axis Vector"=w65) -> ("Rotation3d"=w12:T1)  [unwired: 9 in]
  n285 = call <vilib>:"Quaternion_Get_All.vi"("Quaternion"=w122) -> ("Z"=w112:dbl, "Y"=w113:dbl, "X"=w114:dbl, "W"=w121:dbl)  [unwired: 7 in]
  n286 = call <vilib>:"Rotation3d_Create_AxisAngle.vi"("Angle"=w379, "Axis Vector"=w332) -> ("Rotation3d"=w373:T1)  [unwired: 9 in]
  n287 = call <vilib>:"Rotation3d_Create_AxisAngle.vi"("Angle"=w377, "Axis Vector"=w332) -> ("Rotation3d"=w372:T1)  [unwired: 9 in]
  n288 = call <vilib>:"Quaternion_Get_All.vi"("Quaternion"=w148) -> ("Z"=w138:dbl, "Y"=w139:dbl, "X"=w140:dbl, "W"=w147:dbl)  [unwired: 7 in]
  n289 = Not(x=w452) -> (.not. x?=w451:bool)
  n290 = call <vilib>:"Quaternion_Get_All.vi"("Quaternion"=w97) -> ("Z"=w87:dbl, "Y"=w88:dbl, "X"=w89:dbl, "W"=w96:dbl)  [unwired: 7 in]
  n291 = call <vilib>:"Rotation3d_Create_AxisAngle.vi"("Angle"=w354, "Axis Vector"=w332) -> ("Rotation3d"=w348:T1)  [unwired: 9 in]
  n292 = call <vilib>:"Rotation3d_Create_AxisAngle.vi"("Angle"=w352, "Axis Vector"=w332) -> ("Rotation3d"=w347:T1)  [unwired: 9 in]
  n293 = call <vilib>:"Rotation3d_GetAxisAngle.vi"("in Rotation3d"=w514) -> ("Angle"=w509:dbl, "Axis Vector"=w513:dbl[])  [unwired: 9 in]
  n294 = call <vilib>:"Rotation3d_GetAxisAngle.vi"("in Rotation3d"=w503) -> ("Angle"=w499:dbl, "Axis Vector"=w502:dbl[])  [unwired: 9 in]
  n295 = call <vilib>:"Rotation3d_Create_AxisAngle.vi"("Angle"=w314, "Axis Vector"=w255) -> ("Rotation3d"=w308:T1)  [unwired: 9 in]
  n296 = call <vilib>:"Rotation3d_Create_AxisAngle.vi"("Angle"=w312, "Axis Vector"=w255) -> ("Rotation3d"=w307:T1)  [unwired: 9 in]
  n297 = call <vilib>:"Rotation3d_GetAxisAngle.vi"("in Rotation3d"=w496) -> ("Angle"=w492:dbl, "Axis Vector"=w495:dbl[])  [unwired: 9 in]
  n298 = call <vilib>:"Rotation3d_Create_RollPitchYaw.vi"("Yaw"=w64, "Pitch"=w63, "Roll"=w62) -> ("Rotation3d"=w58:T1)  [unwired: 8 in]
  n299 = call <vilib>:"Rotation3d_Create_AxisAngle.vi"("Angle"=w289, "Axis Vector"=w255) -> ("Rotation3d"=w283:T1)  [unwired: 9 in]
  n300 = call <vilib>:"Rotation3d_Create_AxisAngle.vi"("Angle"=w287, "Axis Vector"=w255) -> ("Rotation3d"=w282:T1)  [unwired: 9 in]
  n301 = Compound Arithmetic op=AND(w528, w527) -> (w526:bool)
  n302 = And(x=w211, y=w210) -> (x .and. y?=w190:bool)
  n303 = Multiply(x=1.5707963267948966, y=0.5) -> (x*y=w487:dbl)
  n304 = call-poly <vilib>:"Array To Matrix.vi"("Real 1D Array"=w512) -> ("Real Matrix (Column Vector)"=w511:T3)
  n305 = call-poly <vilib>:"Array To Matrix.vi"("Real 1D Array"=w491) -> ("Real Matrix (Column Vector)"=w501:T3)
  n306 = call-poly <vilib>:"Array To Matrix.vi"("Real 1D Array"=w513) -> ("Real Matrix (Column Vector)"=w510:T3)
  n307 = call-poly <vilib>:"Array To Matrix.vi"("Real 1D Array"=w502) -> ("Real Matrix (Column Vector)"=w500:T3)
  n308 = call-poly <vilib>:"Array To Matrix.vi"("Real 1D Array"=w490) -> ("Real Matrix (Column Vector)"=w494:T3)
  n309 = call-poly <vilib>:"Array To Matrix.vi"("Real 1D Array"=w495) -> ("Real Matrix (Column Vector)"=w493:T3)
  n310 = Divide(x=3.141592653589793, y=3.0) -> (x/y=w482:dbl)
  n311 = Multiply(x=w114, y=w104) -> (x*y=w111:dbl)
  n312 = Multiply(x=w113, y=w103) -> (x*y=w110:dbl)
  n313 = Multiply(x=w112, y=w102) -> (x*y=w109:dbl)
  n314 = Multiply(x=w140, y=w129) -> (x*y=w137:dbl)
  n315 = Multiply(x=w139, y=w128) -> (x*y=w136:dbl)
  n316 = Multiply(x=w138, y=w127) -> (x*y=w135:dbl)
  n317 = Multiply(x=w89, y=w79) -> (x*y=w86:dbl)
  n318 = Multiply(x=w88, y=w78) -> (x*y=w85:dbl)
  n319 = Multiply(x=w87, y=w77) -> (x*y=w84:dbl)
  n320 = Compound Arithmetic op=AND(w791, w790, w789) -> (w783:bool)
  n321 = Compound Arithmetic op=AND(w772, w771, w770) -> (w764:bool)
  n322 = Compound Arithmetic op=AND(w755, w754, w753) -> (w749:bool)
  n323 = Compound Arithmetic op=AND(w741, w740, w739) -> (w735:bool)
  n324 = call <vilib>:"Util_ApproxEquals.vi"("Value 2"=1.5707963267948966, "Value 1"=w509) -> ("ApproxEquals"=w506:bool)  [unwired: 9 in]
  n325 = call <vilib>:"Matrix_IsEqual.vi"("other"=w510, "input matrix"=w511) -> ("Equal"=w507:bool)  [unwired: 9 in]
  n326 = call <vilib>:"Util_ApproxEquals.vi"("Value 2"=w487, "Value 1"=w499) -> ("ApproxEquals"=w485:bool)  [unwired: 9 in]
  n327 = call <vilib>:"Matrix_IsEqual.vi"("other"=w500, "input matrix"=w501) -> ("Equal"=w486:bool)  [unwired: 9 in]
  n328 = call <vilib>:"Util_ApproxEquals.vi"("Value 2"=0.0, "Value 1"=w121) -> ("ApproxEquals"=w115:bool)  [unwired: 9 in]
  n329 = call <vilib>:"Util_ApproxEquals.vi"("Value 2"=0.0, "Value 1"=w147) -> ("ApproxEquals"=w141:bool)  [unwired: 9 in]
  n330 = call <vilib>:"Util_ApproxEquals.vi"("Value 2"=w482, "Value 1"=w492) -> ("ApproxEquals"=w480:bool)  [unwired: 9 in]
  n331 = call <vilib>:"Matrix_IsEqual.vi"("other"=w493, "input matrix"=w494) -> ("Equal"=w481:bool)  [unwired: 9 in]
  n332 = call <vilib>:"Util_ApproxEquals.vi"("Value 2"=0.0, "Value 1"=w96) -> ("ApproxEquals"=w90:bool)  [unwired: 9 in]
  n333 = Compound Arithmetic op=AND(w717, w701, w689, w680) -> (w679:bool)
  n334 = call <vilib>:"Rotation3d_Interpolate.vi"("T"=0.25, "EndValue Rotation3d"=w433, "in Rotation3d"=w434) -> ("Interpolated Rotation3d"=w421:T1)  [unwired: 8 in]
  n335 = call <vilib>:"Rotation3d_Interpolate.vi"("T"=0.5, "EndValue Rotation3d"=w433, "in Rotation3d"=w434) -> ("Interpolated Rotation3d"=w424:T1)  [unwired: 8 in]
  n336 = call <vilib>:"Rotation3d_Interpolate.vi"("T"=0.25, "EndValue Rotation3d"=w403, "in Rotation3d"=w404) -> ("Interpolated Rotation3d"=w391:T1)  [unwired: 8 in]
  n337 = call <vilib>:"Rotation3d_Interpolate.vi"("T"=0.75, "EndValue Rotation3d"=w433, "in Rotation3d"=w434) -> ("Interpolated Rotation3d"=w418:T1)  [unwired: 8 in]
  n338 = call <vilib>:"Rotation3d_Interpolate.vi"("T"=0.5, "EndValue Rotation3d"=w403, "in Rotation3d"=w404) -> ("Interpolated Rotation3d"=w394:T1)  [unwired: 8 in]
  n339 = call <vilib>:"Rotation3d_Interpolate.vi"("T"=0.25, "EndValue Rotation3d"=w372, "in Rotation3d"=w373) -> ("Interpolated Rotation3d"=w361:T1)  [unwired: 8 in]
  n340 = call <vilib>:"Rotation3d_Interpolate.vi"("T"=0.75, "EndValue Rotation3d"=w403, "in Rotation3d"=w404) -> ("Interpolated Rotation3d"=w388:T1)  [unwired: 8 in]
  n341 = Compound Arithmetic op=ADD(w111, w110, w109) -> (w117:dbl)
  n342 = call <vilib>:"Rotation3d_Interpolate.vi"("T"=0.5, "EndValue Rotation3d"=w372, "in Rotation3d"=w373) -> ("Interpolated Rotation3d"=w364:T1)  [unwired: 8 in]
  n343 = Compound Arithmetic op=ADD(w137, w136, w135) -> (w143:dbl)
  n344 = call <vilib>:"Rotation3d_Equals.vi"("other Rotation3d"=w44, "in Rotation3d"=w11) -> ("Equals"=w30:bool)  [unwired: 9 in]
  n345 = call <vilib>:"Rotation3d_Interpolate.vi"("T"=0.25, "EndValue Rotation3d"=w347, "in Rotation3d"=w348) -> ("Interpolated Rotation3d"=w339:T1)  [unwired: 8 in]
  n346 = call <vilib>:"Rotation3d_Interpolate.vi"("T"=0.75, "EndValue Rotation3d"=w372, "in Rotation3d"=w373) -> ("Interpolated Rotation3d"=w358:T1)  [unwired: 8 in]
  n347 = Compound Arithmetic op=ADD(w86, w85, w84) -> (w92:dbl)
  n348 = call <vilib>:"Rotation3d_Interpolate.vi"("T"=0.5, "EndValue Rotation3d"=w347, "in Rotation3d"=w348) -> ("Interpolated Rotation3d"=w341:T1)  [unwired: 8 in]
  n349 = call <vilib>:"Rotation3d_Equals.vi"("other Rotation3d"=w31, "in Rotation3d"=w10) -> ("Equals"=w29:bool)  [unwired: 9 in]
  n350 = call <vilib>:"Rotation3d_Equals.vi"("other Rotation3d"=w3, "in Rotation3d"=w11) -> ("Equals"=w8:bool)  [unwired: 9 in]
  n351 = call <vilib>:"Rotation3d_Equals.vi"("other Rotation3d"=w1, "in Rotation3d"=w10) -> ("Equals"=w7:bool)  [unwired: 9 in]
  n352 = call <vilib>:"Rotation3d_Interpolate.vi"("T"=0.75, "EndValue Rotation3d"=w347, "in Rotation3d"=w348) -> ("Interpolated Rotation3d"=w336:T1)  [unwired: 8 in]
  n353 = call <vilib>:"Rotation3d_Interpolate.vi"("T"=0.25, "EndValue Rotation3d"=w307, "in Rotation3d"=w308) -> ("Interpolated Rotation3d"=w296:T1)  [unwired: 8 in]
  n354 = call <vilib>:"Rotation3d_Interpolate.vi"("T"=0.5, "EndValue Rotation3d"=w307, "in Rotation3d"=w308) -> ("Interpolated Rotation3d"=w299:T1)  [unwired: 8 in]
  n355 = call <vilib>:"Rotation3d_Interpolate.vi"("T"=0.25, "EndValue Rotation3d"=w282, "in Rotation3d"=w283) -> ("Interpolated Rotation3d"=w274:T1)  [unwired: 8 in]
  n356 = call <vilib>:"Rotation3d_Interpolate.vi"("T"=0.75, "EndValue Rotation3d"=w307, "in Rotation3d"=w308) -> ("Interpolated Rotation3d"=w293:T1)  [unwired: 8 in]
  n357 = call <vilib>:"Rotation3d_Interpolate.vi"("T"=0.5, "EndValue Rotation3d"=w282, "in Rotation3d"=w283) -> ("Interpolated Rotation3d"=w276:T1)  [unwired: 8 in]
  n358 = call <vilib>:"Rotation3d_Interpolate.vi"("T"=0.75, "EndValue Rotation3d"=w282, "in Rotation3d"=w283) -> ("Interpolated Rotation3d"=w271:T1)  [unwired: 8 in]
  n359 = call <vilib>:"Rotation3d_Equals.vi"("other Rotation3d"=w58, "in Rotation3d"=w12) -> ("Equals"=w57:bool)  [unwired: 9 in]
  n360 = Compound Arithmetic op=AND(w783, w764) -> (w763:bool)
  n361 = Compound Arithmetic op=AND(w749, w735) -> (w724:bool)
  n362 = call <vilib>:"Rotation3d_Equals.vi"("other Rotation3d"=w5, "in Rotation3d"=w12) -> ("Equals"=w9:bool)  [unwired: 9 in]
  n363 = call <vilib>:"Util_ApproxEquals.vi"("Value 2"=0.0, "Value 1"=w117) -> ("ApproxEquals"=w116:bool)  [unwired: 9 in]
  n364 = call <vilib>:"Util_ApproxEquals.vi"("Value 2"=0.0, "Value 1"=w143) -> ("ApproxEquals"=w142:bool)  [unwired: 9 in]
  n365 = call <vilib>:"Util_ApproxEquals.vi"("Value 2"=0.0, "Value 1"=w92) -> ("ApproxEquals"=w91:bool)  [unwired: 9 in]
  n366 = Compound Arithmetic op=AND(w507, w506, w486, w485, w481, w480) -> (w479:bool)
  n367 = call <vilib>:"Rotation3d_GetXYZ.vi"("in Rotation3d"=w421) -> ("X"=w417:dbl)  [unwired: 8 in, 2 out]
  n368 = call <vilib>:"Conv_Deg_Radians.vi"("Degress"=55.0) -> ("Radians"=w422:dbl)  [unwired: 10 in]
  n369 = And(x=w115, y=w116) -> (x .and. y?=w73:bool)
  n370 = And(x=w141, y=w142) -> (x .and. y?=w74:bool)
  n371 = call <vilib>:"Rotation3d_GetXYZ.vi"("in Rotation3d"=w424) -> ("Z"=w426:dbl, "Y"=w427:dbl, "X"=w428:dbl)  [unwired: 8 in]
  n372 = call <vilib>:"Rotation3d_GetXYZ.vi"("in Rotation3d"=w391) -> ("X"=w382:dbl)  [unwired: 8 in, 2 out]
  n373 = call <vilib>:"Conv_Deg_Radians.vi"("Degress"=177.5) -> ("Radians"=w392:dbl)  [unwired: 10 in]
  n374 = And(x=w90, y=w91) -> (x .and. y?=w72:bool)
  n375 = call <vilib>:"Rotation3d_GetXYZ.vi"("in Rotation3d"=w418) -> ("X"=w414:dbl)  [unwired: 8 in, 2 out]
  n376 = call <vilib>:"Conv_Deg_Radians.vi"("Degress"=65.0) -> ("Radians"=w419:dbl)  [unwired: 10 in]
  n377 = call <vilib>:"Conv_Deg_Radians.vi"("Degress"=60.0) -> ("Radians"=w415:dbl)  [unwired: 10 in]
  n378 = call <vilib>:"Rotation3d_GetXYZ.vi"("in Rotation3d"=w394) -> ("Z"=w396:dbl, "Y"=w397:dbl, "X"=w398:dbl)  [unwired: 8 in]
  n379 = call <vilib>:"Rotation3d_GetXYZ.vi"("in Rotation3d"=w361) -> ("Y"=w335:dbl)  [unwired: 8 in, 2 out]
  n380 = call <vilib>:"Conv_Deg_Radians.vi"("Degress"=55.0) -> ("Radians"=w362:dbl)  [unwired: 10 in]
  n381 = Compound Arithmetic op=AND(w173, w162, w159, w154, w153, w74, w73, w72) -> (w71:bool)
  "Two Vectors\nTest Passed" <- w71
  n382 = call <vilib>:"Rotation3d_GetXYZ.vi"("in Rotation3d"=w388) -> ("X"=w381:dbl)  [unwired: 8 in, 2 out]
  n383 = call <vilib>:"Conv_Deg_Radians.vi"("Degress"=-167.5) -> ("Radians"=w389:dbl)  [unwired: 10 in]
  n384 = call <vilib>:"Conv_Deg_Radians.vi"("Degress"=-175.0) -> ("Radians"=w386:dbl)  [unwired: 10 in]
  n385 = call <vilib>:"Rotation3d_GetXYZ.vi"("in Rotation3d"=w364) -> ("Z"=w366:dbl, "Y"=w367:dbl, "X"=w368:dbl)  [unwired: 8 in]
  n386 = call <vilib>:"Rotation3d_GetXYZ.vi"("in Rotation3d"=w339) -> ("Y"=w318:dbl)  [unwired: 8 in, 2 out]
  n387 = call <vilib>:"Conv_Deg_Radians.vi"("Degress"=2.5) -> ("Radians"=w319:dbl)  [unwired: 10 in]
  n388 = call <vilib>:"Rotation3d_GetXYZ.vi"("in Rotation3d"=w358) -> ("Y"=w334:dbl)  [unwired: 8 in, 2 out]
  n389 = call <vilib>:"Conv_Deg_Radians.vi"("Degress"=65.0) -> ("Radians"=w359:dbl)  [unwired: 10 in]
  n390 = call <vilib>:"Conv_Deg_Radians.vi"("Degress"=0.0) -> ("Radians"=w326:dbl)  [unwired: 10 in]
  n391 = call <vilib>:"Conv_Deg_Radians.vi"("Degress"=60.0) -> ("Radians"=w327:dbl)  [unwired: 10 in]
  n392 = call <vilib>:"Conv_Deg_Radians.vi"("Degress"=0.0) -> ("Radians"=w328:dbl)  [unwired: 10 in]
  n393 = call <vilib>:"Rotation3d_GetXYZ.vi"("in Rotation3d"=w341) -> ("Z"=w342:dbl, "Y"=w331:dbl, "X"=w343:dbl)  [unwired: 8 in]
  n394 = call <vilib>:"Conv_Deg_Radians.vi"("Degress"=180.0) -> ("Radians"=w322:dbl)  [unwired: 10 in]
  n395 = call <vilib>:"Conv_Deg_Radians.vi"("Degress"=-5.0) -> ("Radians"=w321:dbl)  [unwired: 10 in]
  n396 = call <vilib>:"Conv_Deg_Radians.vi"("Degress"=180.0) -> ("Radians"=w320:dbl)  [unwired: 10 in]
  n397 = call <vilib>:"Rotation3d_GetXYZ.vi"("in Rotation3d"=w336) -> ("Y"=w333:dbl)  [unwired: 8 in, 2 out]
  n398 = call <vilib>:"Conv_Deg_Radians.vi"("Degress"=-12.5) -> ("Radians"=w337:dbl)  [unwired: 10 in]
  n399 = call <vilib>:"Rotation3d_GetXYZ.vi"("in Rotation3d"=w296) -> ("Z"=w254:dbl)  [unwired: 8 in, 2 out]
  n400 = call <vilib>:"Conv_Deg_Radians.vi"("Degress"=55.0) -> ("Radians"=w297:dbl)  [unwired: 10 in]
  n401 = call <vilib>:"Rotation3d_GetXYZ.vi"("in Rotation3d"=w299) -> ("Z"=w301:dbl, "Y"=w302:dbl, "X"=w303:dbl)  [unwired: 8 in]
  n402 = call <vilib>:"Rotation3d_GetXYZ.vi"("in Rotation3d"=w274) -> ("Z"=w252:dbl)  [unwired: 8 in, 2 out]
  n403 = call <vilib>:"Conv_Deg_Radians.vi"("Degress"=177.5) -> ("Radians"=w258:dbl)  [unwired: 10 in]
  n404 = call <vilib>:"Rotation3d_GetXYZ.vi"("in Rotation3d"=w293) -> ("Z"=w253:dbl)  [unwired: 8 in, 2 out]
  n405 = call <vilib>:"Conv_Deg_Radians.vi"("Degress"=65.0) -> ("Radians"=w294:dbl)  [unwired: 10 in]
  n406 = call <vilib>:"Conv_Deg_Radians.vi"("Degress"=0.0) -> ("Radians"=w265:dbl)  [unwired: 10 in]
  n407 = call <vilib>:"Conv_Deg_Radians.vi"("Degress"=0.0) -> ("Radians"=w266:dbl)  [unwired: 10 in]
  n408 = call <vilib>:"Conv_Deg_Radians.vi"("Degress"=60.0) -> ("Radians"=w267:dbl)  [unwired: 10 in]
  n409 = call <vilib>:"Rotation3d_GetXYZ.vi"("in Rotation3d"=w276) -> ("Z"=w277:dbl, "Y"=w270:dbl, "X"=w278:dbl)  [unwired: 8 in]
  n410 = call <vilib>:"Conv_Deg_Radians.vi"("Degress"=0.0) -> ("Radians"=w261:dbl)  [unwired: 10 in]
  n411 = call <vilib>:"Conv_Deg_Radians.vi"("Degress"=0.0) -> ("Radians"=w260:dbl)  [unwired: 10 in]
  n412 = call <vilib>:"Conv_Deg_Radians.vi"("Degress"=-175.0) -> ("Radians"=w259:dbl)  [unwired: 10 in]
  n413 = call <vilib>:"Rotation3d_GetXYZ.vi"("in Rotation3d"=w271) -> ("Z"=w251:dbl)  [unwired: 8 in, 2 out]
  n414 = call <vilib>:"Conv_Deg_Radians.vi"("Degress"=-167.5) -> ("Radians"=w272:dbl)  [unwired: 10 in]
  n415 = call <vilib>:"Util_ApproxEquals.vi"("Value 2"=w422, "Value 1"=w417) -> ("ApproxEquals"=w413:bool)  [unwired: 9 in]
  n416 = call <vilib>:"Util_ApproxEquals.vi"("Value 2"=w392, "Value 1"=w382) -> ("ApproxEquals"=w385:bool)  [unwired: 9 in]
  n417 = call <vilib>:"Util_ApproxEquals.vi"("Value 2"=0.0, "Value 1"=w427) -> ("ApproxEquals"=w430:bool)  [unwired: 9 in]
  n418 = call <vilib>:"Util_ApproxEquals.vi"("Value 2"=0.0, "Value 1"=w426) -> ("ApproxEquals"=w429:bool)  [unwired: 9 in]
  n419 = call <vilib>:"Util_ApproxEquals.vi"("Value 2"=w415, "Value 1"=w428) -> ("ApproxEquals"=w431:bool)  [unwired: 9 in]
  n420 = call <vilib>:"Util_ApproxEquals.vi"("Value 2"=w419, "Value 1"=w414) -> ("ApproxEquals"=w412:bool)  [unwired: 9 in]
  n421 = call <vilib>:"Util_ApproxEquals.vi"("Value 2"=w362, "Value 1"=w335) -> ("ApproxEquals"=w357:bool)  [unwired: 9 in]
  n422 = call <vilib>:"Util_ApproxEquals.vi"("Value 2"=0.0, "Value 1"=w397) -> ("ApproxEquals"=w400:bool)  [unwired: 9 in]
  n423 = call <vilib>:"Util_ApproxEquals.vi"("Value 2"=0.0, "Value 1"=w396) -> ("ApproxEquals"=w399:bool)  [unwired: 9 in]
  n424 = call <vilib>:"Util_ApproxEquals.vi"("Value 2"=w386, "Value 1"=w398) -> ("ApproxEquals"=w401:bool)  [unwired: 9 in]
  n425 = call <vilib>:"Util_ApproxEquals.vi"("Value 2"=w389, "Value 1"=w381) -> ("ApproxEquals"=w384:bool)  [unwired: 9 in]
  n426 = call <vilib>:"Util_ApproxEquals.vi"("Value 2"=w319, "Value 1"=w318) -> ("ApproxEquals"=w317:bool)  [unwired: 9 in]
  n427 = call <vilib>:"Util_ApproxEquals.vi"("Value 2"=w327, "Value 1"=w367) -> ("ApproxEquals"=w370:bool)  [unwired: 9 in]
  n428 = call <vilib>:"Util_ApproxEquals.vi"("Value 2"=w328, "Value 1"=w366) -> ("ApproxEquals"=w369:bool)  [unwired: 9 in]
  n429 = call <vilib>:"Util_ApproxEquals.vi"("Value 2"=w326, "Value 1"=w368) -> ("ApproxEquals"=w371:bool)  [unwired: 9 in]
  n430 = call <vilib>:"Util_ApproxEquals.vi"("Value 2"=w359, "Value 1"=w334) -> ("ApproxEquals"=w356:bool)  [unwired: 9 in]
  n431 = Compound Arithmetic op=AND(w57, w30, w29, w9, w8, w7) -> (w28:bool)
  "Axis Angle\nTest Passed" <- w28
  n432 = call <vilib>:"Util_ApproxEquals.vi"("Value 2"=w321, "Value 1"=w331) -> ("ApproxEquals"=w345:bool)  [unwired: 9 in]
  n433 = call <vilib>:"Util_ApproxEquals.vi"("Value 2"=w320, "Value 1"=w342) -> ("ApproxEquals"=w344:bool)  [unwired: 9 in]
  n434 = call <vilib>:"Util_ApproxEquals.vi"("Value 2"=w322, "Value 1"=w343) -> ("ApproxEquals"=w346:bool)  [unwired: 9 in]
  n435 = call <vilib>:"Util_ApproxEquals.vi"("Value 2"=w337, "Value 1"=w333) -> ("ApproxEquals"=w316:bool)  [unwired: 9 in]
  n436 = call <vilib>:"Util_ApproxEquals.vi"("Value 2"=w297, "Value 1"=w254) -> ("ApproxEquals"=w292:bool)  [unwired: 9 in]
  n437 = call <vilib>:"Util_ApproxEquals.vi"("Value 2"=w258, "Value 1"=w252) -> ("ApproxEquals"=w257:bool)  [unwired: 9 in]
  n438 = call <vilib>:"Util_ApproxEquals.vi"("Value 2"=w266, "Value 1"=w302) -> ("ApproxEquals"=w305:bool)  [unwired: 9 in]
  n439 = call <vilib>:"Util_ApproxEquals.vi"("Value 2"=w267, "Value 1"=w301) -> ("ApproxEquals"=w304:bool)  [unwired: 9 in]
  n440 = call <vilib>:"Util_ApproxEquals.vi"("Value 2"=w265, "Value 1"=w303) -> ("ApproxEquals"=w306:bool)  [unwired: 9 in]
  n441 = call <vilib>:"Util_ApproxEquals.vi"("Value 2"=w294, "Value 1"=w253) -> ("ApproxEquals"=w291:bool)  [unwired: 9 in]
  n442 = call <vilib>:"Util_ApproxEquals.vi"("Value 2"=w260, "Value 1"=w270) -> ("ApproxEquals"=w280:bool)  [unwired: 9 in]
  n443 = call <vilib>:"Util_ApproxEquals.vi"("Value 2"=w259, "Value 1"=w277) -> ("ApproxEquals"=w279:bool)  [unwired: 9 in]
  n444 = call <vilib>:"Util_ApproxEquals.vi"("Value 2"=w261, "Value 1"=w278) -> ("ApproxEquals"=w281:bool)  [unwired: 9 in]
  n445 = call <vilib>:"Util_ApproxEquals.vi"("Value 2"=w272, "Value 1"=w251) -> ("ApproxEquals"=w256:bool)  [unwired: 9 in]
  n446 = Compound Arithmetic op=AND(w413, w431, w430, w429, w412) -> (w250:bool)
  n447 = Compound Arithmetic op=AND(w385, w401, w400, w399, w384) -> (w249:bool)
  n448 = Compound Arithmetic op=AND(w357, w371, w370, w369, w356) -> (w248:bool)
  n449 = Compound Arithmetic op=AND(w190, w189, w188) -> (→"Rot Mat\nTest Passed":bool)
  n450 = Compound Arithmetic op=AND(w317, w346, w345, w344, w316) -> (w247:bool)
  n451 = Compound Arithmetic op=AND(w292, w306, w305, w304, w291) -> (w246:bool)
  n452 = Compound Arithmetic op=AND(w257, w281, w280, w279, w256) -> (w245:bool)
  n453 = Compound Arithmetic op=AND(w250, w249, w248, w247, w246, w245) -> (w244:bool)
  n454 = Compound Arithmetic op=AND(w806, w763, w724, w679, w669, w659, w649, w626, w603, w580, w557, w526, w479, w467, w451, w244, w190, w189, w188, w71, w28) -> (→"ALL TESTS PASSED":bool)
  "error out" <- "error in (no error)"
